vi "main 0.7.vi"() -> ()   [LabVIEW 2012]
uses:
  coherent/CH_LM/CH_LM Communication Mode.ctl
  ISEGNHQxxu/iseg NHQ VISA Control.ctl
  <vilib>/Utility/file.llb/Read From Spreadsheet File (DBL).vi
  <vilib>/Analysis/1siggen.llb/Ramp Pattern by Samples.vi
  <vilib>/Utility/file.llb/Write To Spreadsheet File (DBL).vi
  <vilib>/Utility/file.llb/Write To Spreadsheet File (string).vi
  <vilib>/Platform/browser.llb/Open URL in Default Browser (path).vi
  <vilib>/Analysis/NI_AALBase.lvlib
  coherent/CH_LM.lvlib
panel:
  in  "array size":i32
  out "power noise-o-meter":dbl format="%.1g"
  out "power history":dbl(graph)
  out "signal noise-o-meter":dbl format="%.1g"
  in  "Nominal Voltage":sgl=50.0 max=4000 format="%.2f"
  in  "volt_set":bool
  in  "open base path":bool
  out "laser power":sgl=6.5658234e-09 format="%^#_3e"
  out "Actual Voltage":dbl=-50.050000000000004 format="%.2f"
  out "Waveform Chart":dbl(graph)
  in  "Path":path=path "Y:/Ediff/data/2016/10/161018"
  in  "stop":bool
  out "Slide":dbl(slide)=0.999 scale=0.0..1.0
  in  "Tab Control":T1(tab)
  in  "savepng":bool
  in  "savebin":bool
  in  "dark_load":bool
  in  "binning":dbl=4.0
  in  "exp time [s]":dbl=0.01
  in  "frames":i32=1000
  in  "avg[t] acc[f]":bool=TRUE
  in  "threshold":i32=110
  in  "dark?":bool=TRUE
  in  "dark":bool
  in  "snap":bool
  in  "count?":bool
  in  "move2com":bool
  in  "window2":dbl=10000.0 caption="+/- window" format="%#_6e"
  in  "steps2":u32=21 caption="steps"
  out "XY":dbl[][](graph)
  in  "meas_start_XY":bool
  in  "Axis2":string(combo)="4D Z"
  in  "Axis1":string(combo)="4D Z"
  in  "window1":dbl=10000.0 caption="+/- window" format="%#_6e"
  in  "steps1":u32=21 caption="steps"
  in  "meas_stop_XY":bool
  in  "showcom":bool
  out "Slide 2":dbl(slide)=0.999 scale=0.0..1.0
  in  "meas_stop_volt":bool
  in  "meas_start_volt":bool
  in  "head":string="PowerVoltScan1"
  in  "volt_start":dbl format="%0.2f"
  in  "volt_end":dbl=1.0 format="%0.2f"
  in  "volt_samples":i32=128
  out "Boolean":bool
  out "XY Graph":cluster{sgl[], dbl[]}(graph)
  in  "x .or. y?":bool
  in  "head 2":string="PowerVoltScan1"
  in  "meas_start_power":bool
  in  "VISA ISEG":refnum<visa-resource-name>="COM6"
  in  "Channel (A)":enum16{"A", "B"}(ring)=enum."B"
  in  "IP address":string="172.24.192.135"
  out "error out":errorcluster
  out "coherent":errorcluster
  in  "volt_timeout":u32=6000
  in  "volt_threshold":sgl=2.0 max=4000 format="%.2f"
  out "captured":dbl[][](graph)
  out "live":dbl[][](graph)
  in  "close":bool
  # "%"
  # "%"
  # "V"
  # "W"
  # "Axis2"
  # "Axis1"
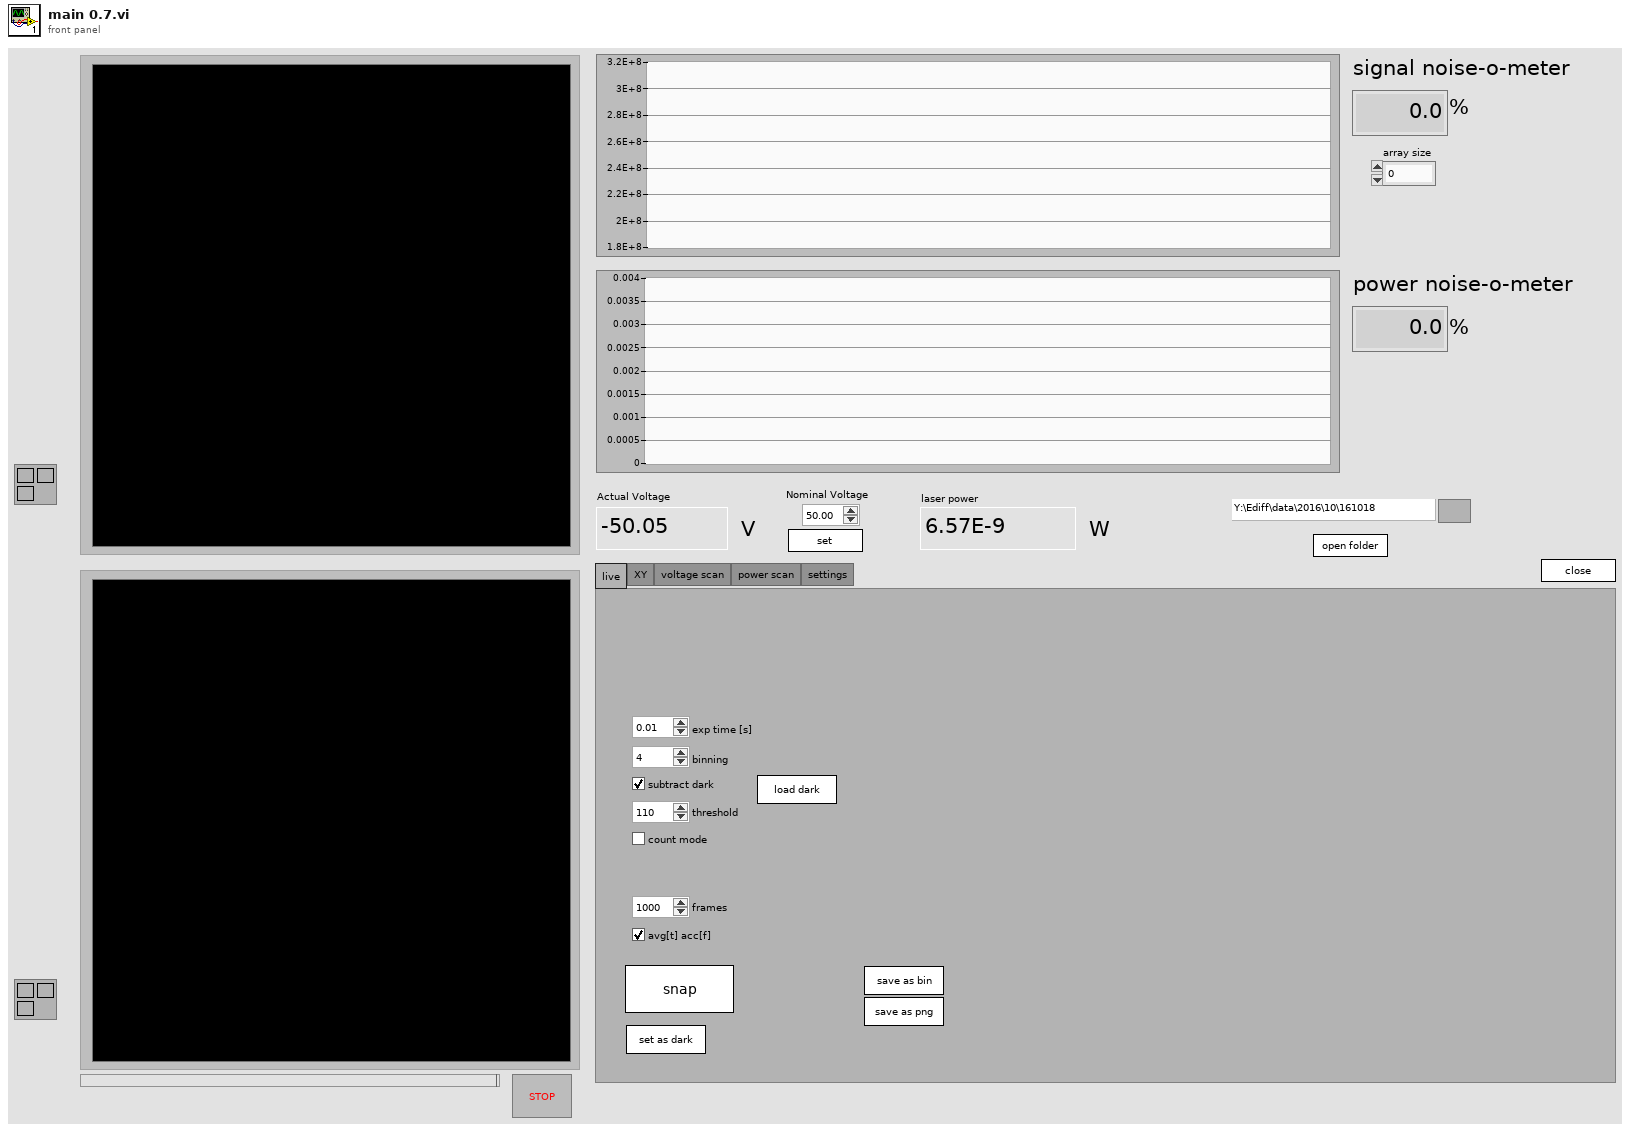
[diagram p1: front panel]
types:
  T1 = enum32{"live", "XY", "voltage scan", "power scan", "settings"}
  T2 = typedef "CH_LM.lvlib/CH_LM Communication Mode.ctl" = enum16{"None", "USB", "GPIB", "RS232"}
  T3 = typedef "Image Type" = u32
  T4 = typedef "IMAQ Image.ctl" = refnum<image>
  T5 = cluster{"height":u32, "width":u32, "datatype":u32}
  T6 = typedef "iseg NHQ VISA Control.ctl" = cluster{"VISA Resource Name":refnum<visa-resource-name>, "FP Notation":bool, "Maximum Voltage":u32, "Maximum Current":u32}
  T7 = typedef "CH_LM.lvlib/CH_LM Streaming Data.ctl" = cluster{"Value":sgl, "Quad Distance":cluster{"X":sgl, "Y":sgl}, "Display Data":cluster{"Format ID":u8, "Scale ID":u8}, "Unit ID":u8, "Flags":u32, "Pulse Period":u32, "Sequence ID":u32, "Unit String":string}
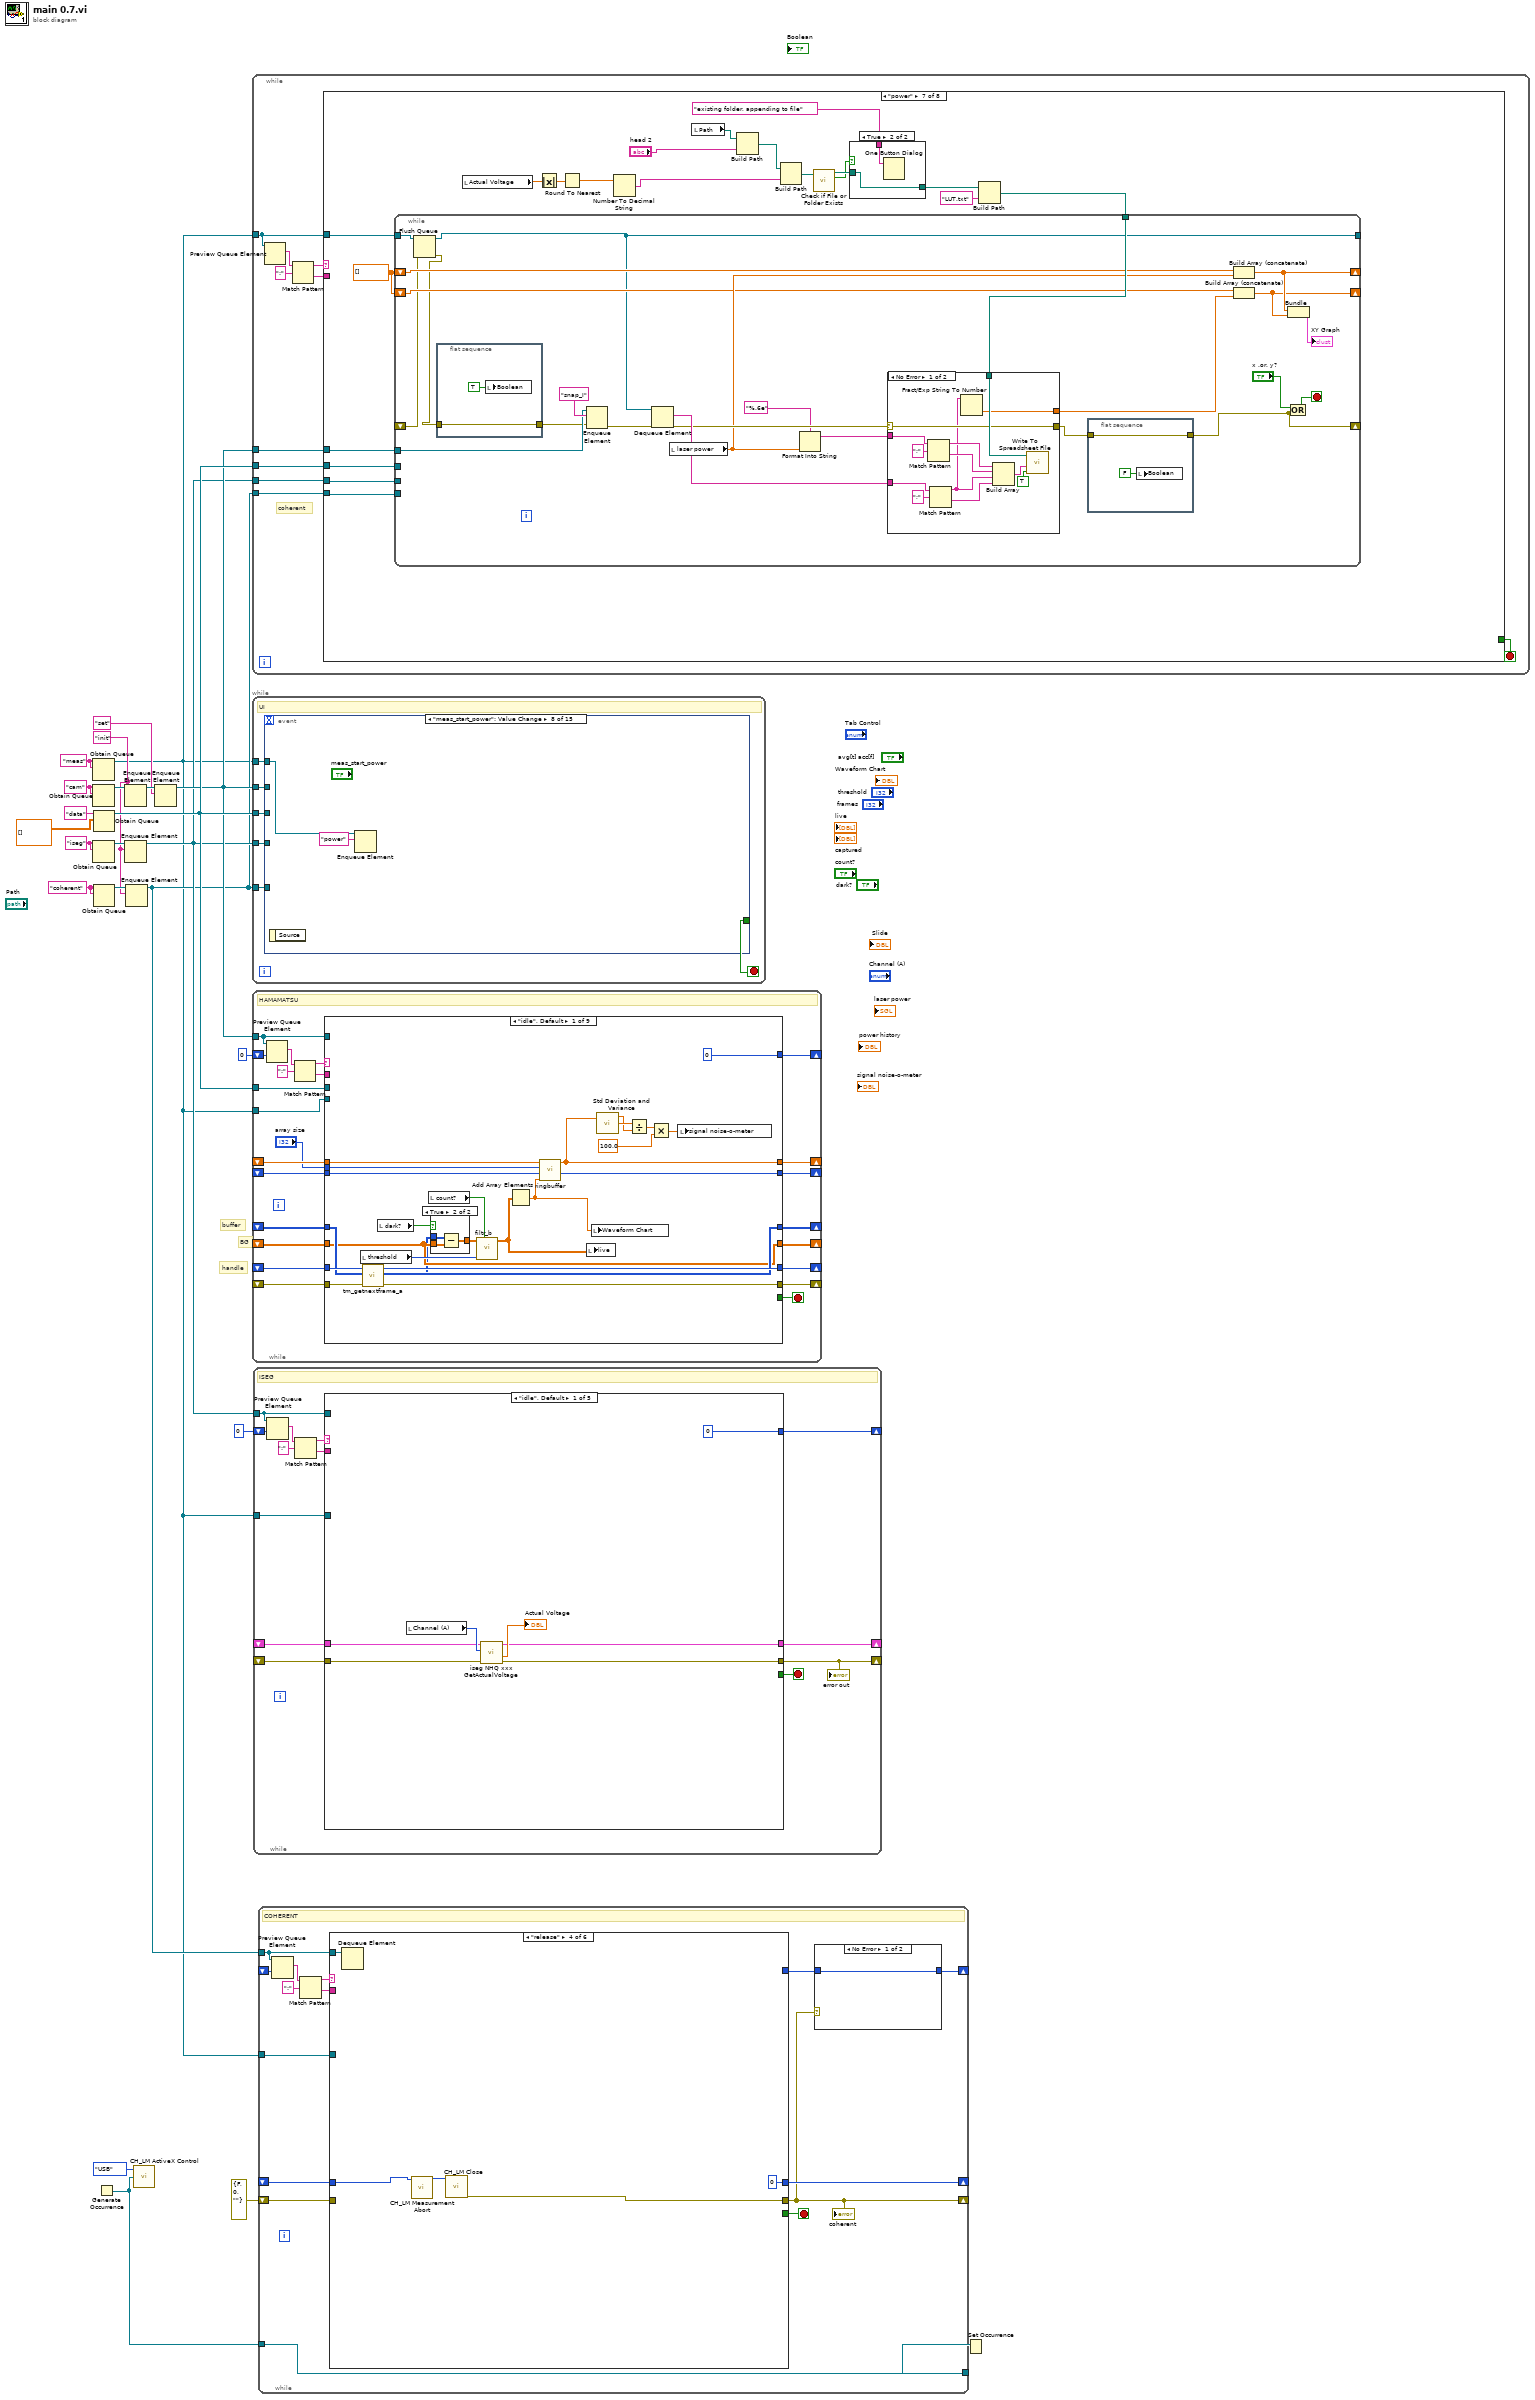
[diagram p0: block diagram]
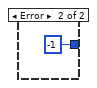
[diagram p2: hidden frame]
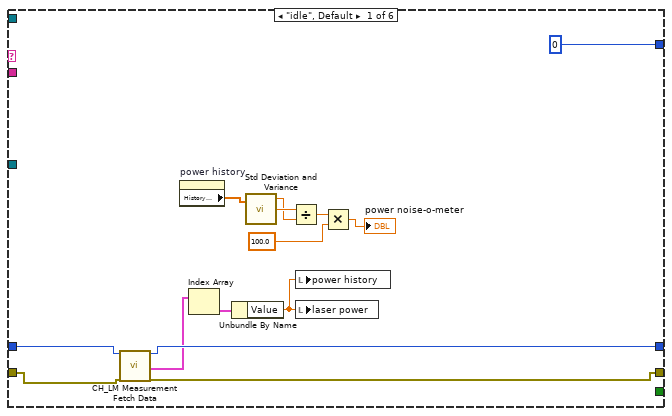
[diagram p3: hidden frame]
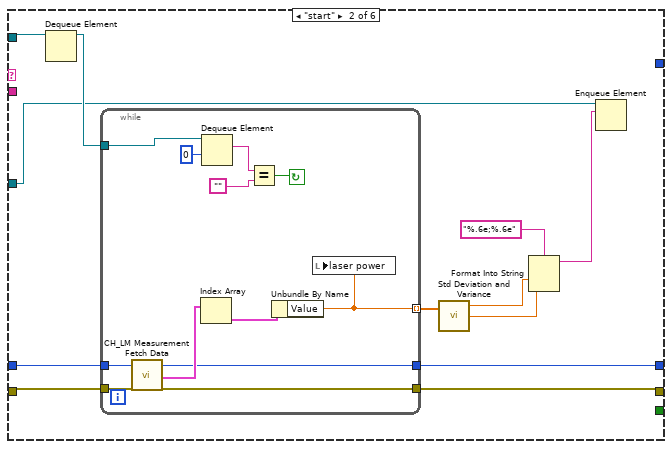
[diagram p4: hidden frame]
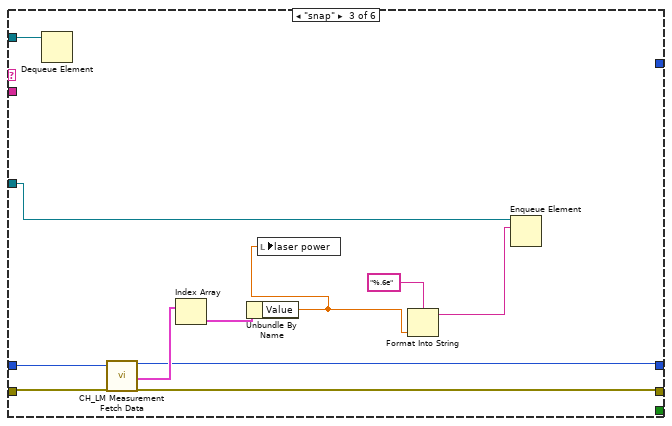
[diagram p5: hidden frame]
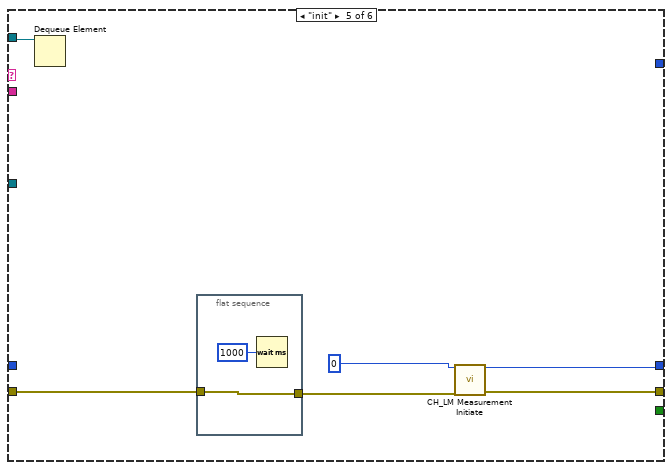
[diagram p6: hidden frame]
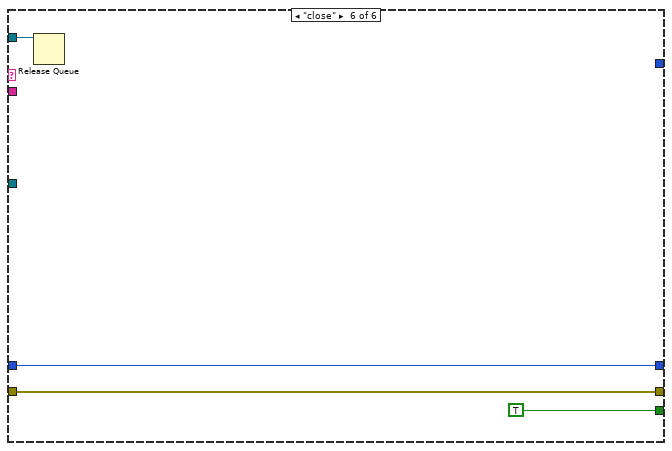
[diagram p7: hidden frame]
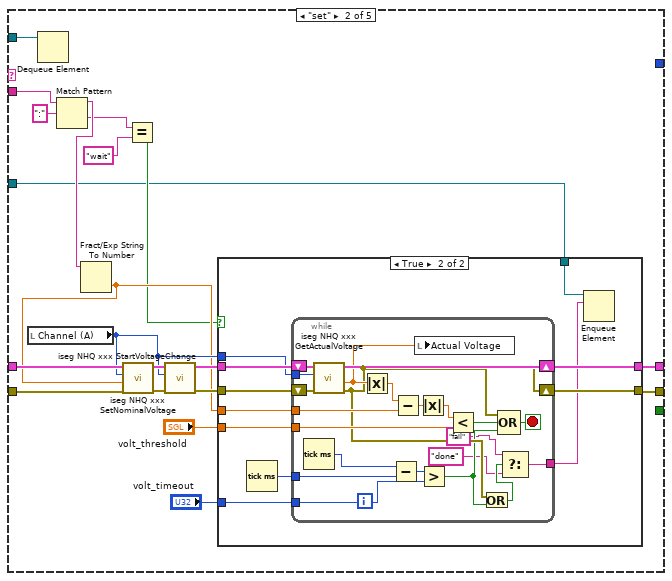
[diagram p8: hidden frame]
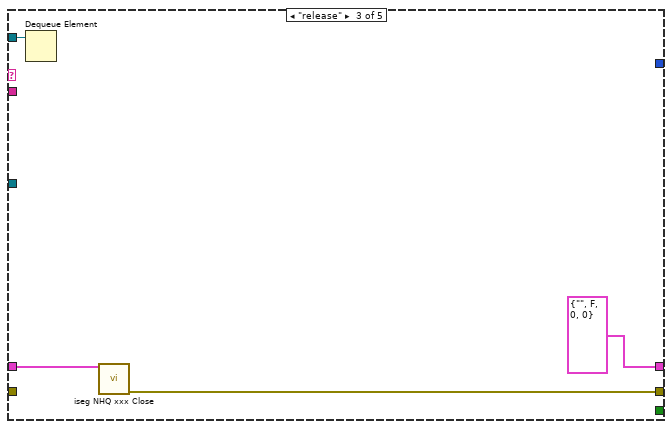
[diagram p10: hidden frame]
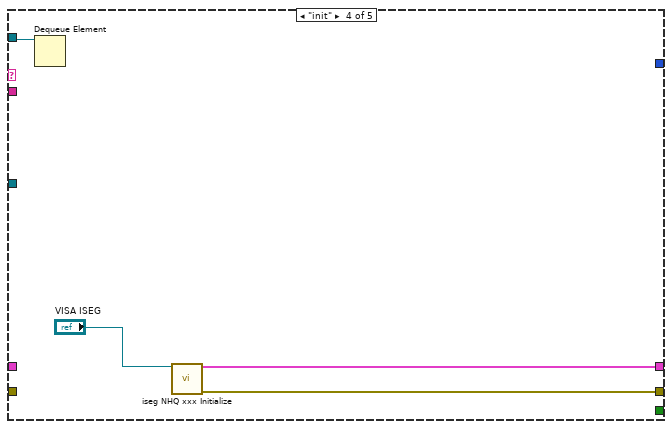
[diagram p11: hidden frame]
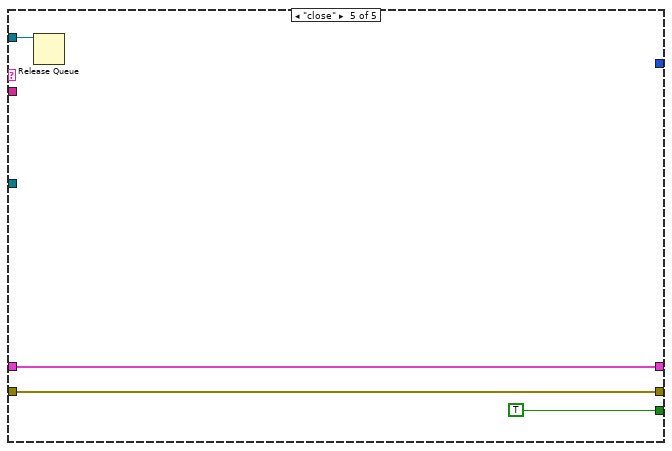
[diagram p12: hidden frame]
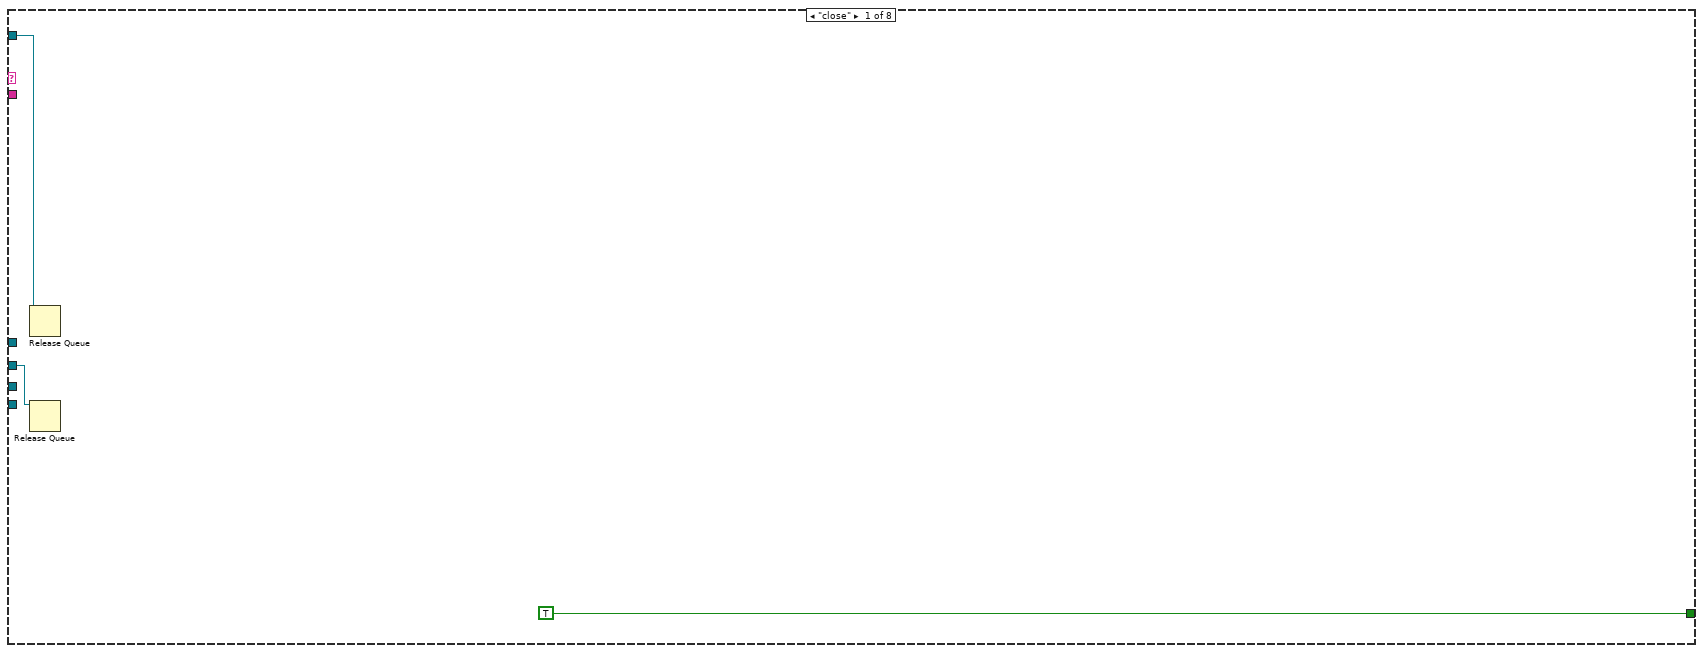
[diagram p13: hidden frame]
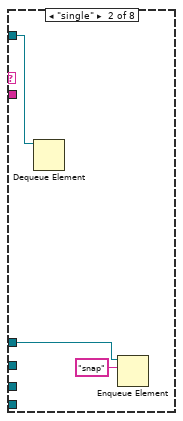
[diagram p14: hidden frame]
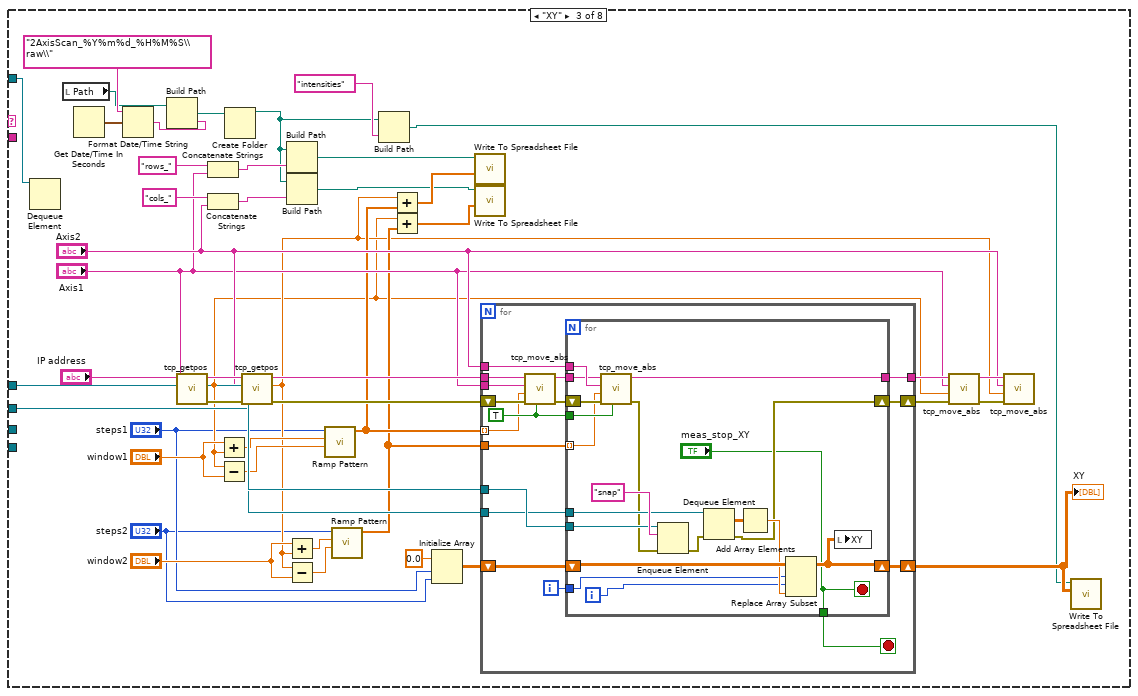
[diagram p15: hidden frame]
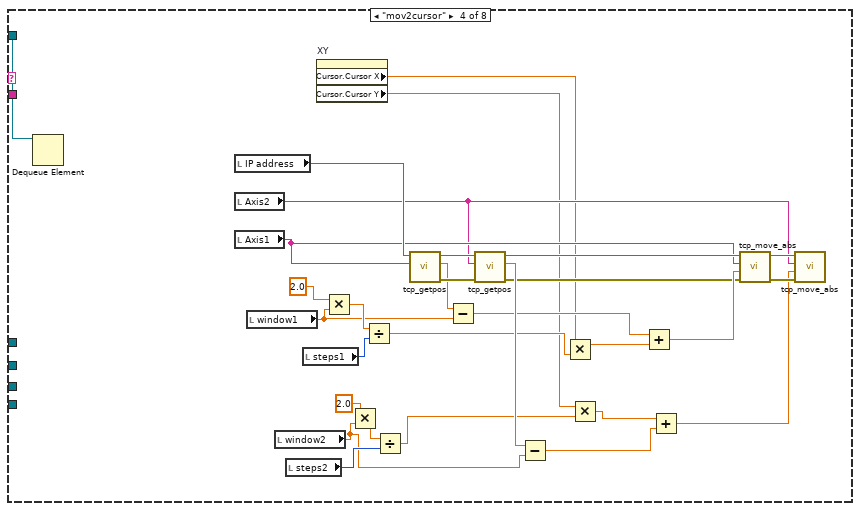
[diagram p16: hidden frame]
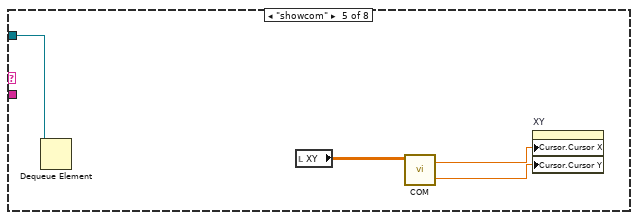
[diagram p17: hidden frame]
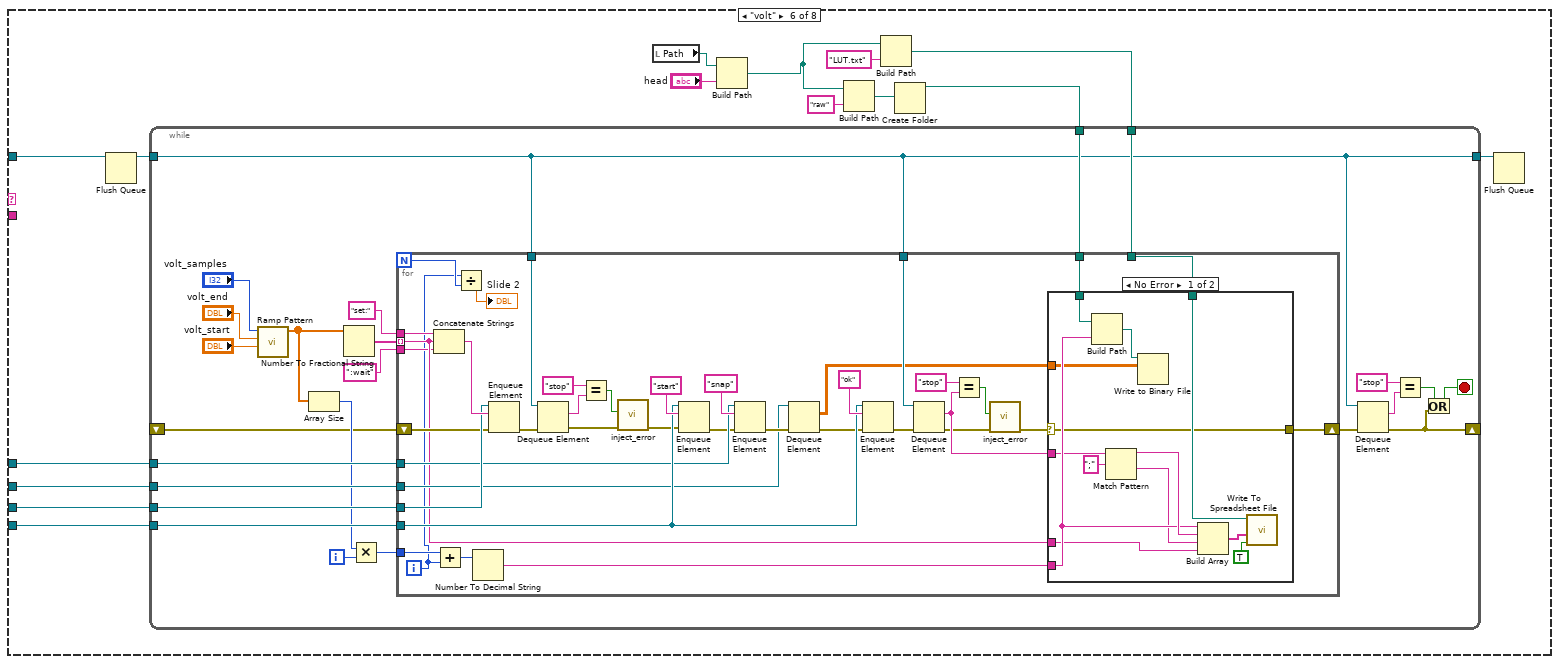
[diagram p18: hidden frame]
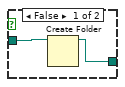
[diagram p20: hidden frame]
diagram:
  w8 = "coherent" ("name (unnamed)")
  w13 = "iseg" ("name (unnamed)")
  w7 = "init" ("element")
  w20 = "meas" ("name (unnamed)")
  w21 = "cam" ("name (unnamed)")
  # "BG"
  # "handle"
  # "buffer"
  n1 = Obtain Queue(name (unnamed)=w20, element data type=w20) -> (queue out=w1:refnum<queue>)  [unwired: 3 in, 2 out]
  n2 = Obtain Queue(name (unnamed)=w21, element data type=w21) -> (queue out=w23:refnum<queue>)  [unwired: 3 in, 2 out]
  n3 = Obtain Queue(name (unnamed)=w13, element data type=w13) -> (queue out=w12:refnum<queue>)  [unwired: 3 in, 2 out]
  n4 = Obtain Queue(name (unnamed)="data", element data type=dbl[][] []) -> (queue out=w16:refnum<queue>)  [unwired: 3 in, 2 out]
  n5 = Obtain Queue(name (unnamed)=w8, element data type=w8) -> (queue out=w9:refnum<queue>)  [unwired: 3 in, 2 out]
  n6 = Generate Occurrence() -> (w5:refnum<k4>)
  n7 = Enqueue Element(queue=w23, element=w7) -> (queue out=w19:refnum<queue>)  [unwired: 2 in, 2 out]
  n8 = Enqueue Element(queue=w12, element=w7) -> (queue out=w10:refnum<queue>)  [unwired: 2 in, 2 out]
  n9 = Enqueue Element(queue=w9, element=w7) -> (queue out=w3:refnum<queue>)  [unwired: 2 in, 2 out]
  n10 = call "CH_LM ActiveX Control.vi"("Communication Mode"=CH_LM_Communication_Mode."USB", "MonitorStop Occurrence"=w5) -> ()  [unwired: 3 in, 1 out]
  n11 = Enqueue Element(queue=w19, element="set") -> (queue out=w15:refnum<queue>)  [unwired: 2 in, 2 out]
  n12 = while {
    tunnel: w1 -> [w29]
    tunnel: w16 -> [w28]
    tunnel: w15 -> [w26]
    tunnel: w10 -> [w25]
    tunnel: w3 -> [w24]
    stop <- w27 stop-if-true
    # "coherent"
    n13 = Preview Queue Element(queue=w29) -> (element=w33:string)  [unwired: 2 in, 3 out]
    n14 = Match Pattern(string=w33, regular expression=":") -> (before substring=w31:string, after substring=w30:string)  [unwired: 1 in, 2 out]
    n15 = case shown="\"power\"" w31 {
      tunnel: w30 -> [_ _ _ _ _ _ _ _]
      tunnel: w29 -> [w35 w39 w84 w150 w151 w169 w257 _]
      tunnel: w28 -> [w36 _ w80 _ _ w161 w264 _]
      tunnel: [TRUE _ _ _ _ _ _ _] -> w27
      tunnel: w26 -> [_ w38 w81 _ _ w162 w265 _]
      tunnel: w25 -> [_ _ _ _ _ w163 w263 _]
      tunnel: w24 -> [_ _ _ _ _ w164 w262 _]
      frame "close" {
        n16 = Release Queue(queue=w35) -> ()  [unwired: 2 in, 3 out]
        n17 = Release Queue(queue=w36) -> ()  [unwired: 2 in, 3 out]
      }
      frame "single" {
        n18 = Dequeue Element(queue=w39) -> ()  [unwired: 2 in, 4 out]
        n19 = Enqueue Element(queue=w38, element="snap") -> ()  [unwired: 2 in, 3 out]
      }
      frame "XY" {
        n20 = Dequeue Element(queue=w84) -> ()  [unwired: 2 in, 4 out]
        n21 = local read "Path"() -> (w75:path)
        n22 = Get Date/Time In Seconds() -> (seconds since 1Jan1904=w79:timestamp)
        n23 = Format Date/Time String(time format string (%c)="2AxisScan_%Y%m%d_%H%M%S\\raw\\", seconds (now)=w79) -> (date/time string=w43:string)  [unwired: 1 in]
        n24 = Build Path(base path=w75, name or relative path=w43) -> (appended path=w47:path)
        n25 = call "tcp_getpos.vi"("Axis"="Axis1", "IP address"="IP address") -> ("error out"=w76:errorcluster, "position"=w52:dbl, "IP address out"=w77:string)  [unwired: 7 in]
        n26 = Concatenate Strings("rows_" ("string"), "Axis1") -> (w44:string)
        n27 = Concatenate Strings("cols_" ("string"), "Axis2") -> (w74:string)
        n28 = Add(x="window1", y=w52) -> (x+y=w59:dbl)
        n29 = Subtract(x=w52, y="window1") -> (x-y=w58:dbl)
        n30 = Create Folder(path (use dialog)=w47) -> (created path=w42:path)  [unwired: 2 in, 2 out]
        n31 = call "tcp_getpos.vi"("error in (no error)"=w76, "Axis"="Axis2", "IP address"=w77) -> ("error out"=w69:errorcluster, "position"=w53:dbl, "IP address out"=w64:string)  [unwired: 6 in]
        n32 = Build Path(base path=w42, name or relative path=w44) -> (appended path=w41:path)
        n33 = Build Path(base path=w42, name or relative path=w74) -> (appended path=w40:path)
        n34 = Add(x="window2", y=w53) -> (x+y=w56:dbl)
        n35 = Subtract(x=w53, y="window2") -> (x-y=w57:dbl)
        n36 = call-poly <vilib>:"Ramp Pattern.vi"("start"=w58, "end"=w59, "samples"="steps1") -> ("Ramp Pattern"=w55:dbl[])  [unwired: 7 in, 1 out]
        n37 = call-poly <vilib>:"Ramp Pattern.vi"("start"=w57, "end"=w56, "samples"="steps2") -> ("Ramp Pattern"=w54:dbl[])  [unwired: 7 in, 1 out]
        n38 = Build Path(base path=w42, name or relative path="intensities") -> (appended path=w45:path)
        n39 = Add(x=w53, y=w55) -> (x+y=w51:dbl[])
        n40 = Add(x=w52, y=w54) -> (x+y=w50:dbl[])
        n41 = Initialize Array(0.0 ("element"), "steps1", "steps2") -> (w82:dbl[][])
        n42 = call-poly <vilib>:"Write To Spreadsheet File.vi"("1D data"=w51, "file path (dialog if empty)"=w41) -> ()  [unwired: 6 in, 1 out]
        n43 = call-poly <vilib>:"Write To Spreadsheet File.vi"("1D data"=w50, "file path (dialog if empty)"=w40) -> ()  [unwired: 6 in, 1 out]
        n44 = for {
          tunnel: "Axis1" -> [w101]
          tunnel: w81 -> [w100]
          tunnel: w80 -> [w99]
          tunnel: "Axis2" -> [w95]
          shift-right: [w94] -> w73
          shift-left: w82 -> [w98]
          shift-right: [w91] -> w70
          shift-left: w69 -> [w90]
          tunnel: [w88] -> w65
          tunnel: w64 -> [w87]
          tunnel: w55 -> [w85] mode=indexing
          tunnel: w54 -> [w86]
          i -> [w97]
          stop <- w89 stop-if-true
          w96 = TRUE ("wait4motiondone")
          n45 = call "tcp_move_abs.vi"("wait4motiondone"=w96, "error in (no error)"=w90, "destination nm/u°"=w85, "Axis"=w101, "IP address"=w87) -> ("error out"=w93:errorcluster, "IP address out"=w92:string)  [unwired: 4 in, 1 out]
          n46 = for {
            tunnel: w100 -> [w118]
            tunnel: w99 -> [w117]
            tunnel: w97 -> [w103]
            shift-right: [w108] -> w94
            shift-left: w98 -> [w116]
            tunnel: w96 -> [w112]
            tunnel: w95 -> [w111]
            tunnel: w92 -> [w109]
            shift-right: [w107] -> w91
            shift-left: w93 -> [w110]
            tunnel: ["meas_stop_XY"] -> w89
            tunnel: [w105] -> w88
            tunnel: w86 -> [w104] mode=indexing
            i -> [w102]
            stop <- "meas_stop_XY" stop-if-true
            n47 = call "tcp_move_abs.vi"("wait4motiondone"=w112, "error in (no error)"=w110, "destination nm/u°"=w104, "Axis"=w111, "IP address"=w109) -> ("error out"=w113:errorcluster, "IP address out"=w105:string)  [unwired: 4 in, 1 out]
            n48 = Enqueue Element(queue=w118, element="snap", error in (no error)=w113) -> (error out=w119:errorcluster)  [unwired: 1 in, 2 out]
            n49 = Dequeue Element(queue=w117, error in (no error)=w119) -> (element=w115:dbl[][], error out=w107:errorcluster)  [unwired: 1 in, 2 out]
            n50 = Add Array Elements(numeric array=w115) -> (sum=w114:dbl)
            n51 = Replace Array Subset(array=w116, new element=w114, index (row)=w103, index (col)=w102) -> (w108:dbl[][])
            n52 = local write "XY"(w108) -> ()
          }
        }
        "XY" <- w73
        n53 = call "tcp_move_abs.vi"("error in (no error)"=w70, "destination nm/u°"=w52, "Axis"="Axis1", "IP address"=w65) -> ("error out"=w72:errorcluster, "IP address out"=w71:string)  [unwired: 5 in, 1 out]
        n54 = call "tcp_move_abs.vi"("error in (no error)"=w72, "destination nm/u°"=w53, "Axis"="Axis2", "IP address"=w71) -> ()  [unwired: 5 in, 3 out]
        n55 = call-poly <vilib>:"Write To Spreadsheet File.vi"("2D data"=w73, "file path (dialog if empty)"=w45) -> ()  [unwired: 6 in, 1 out]
      }
      frame "mov2cursor" {
        n56 = Dequeue Element(queue=w150) -> ()  [unwired: 2 in, 4 out]
        n57 = local read "IP address"() -> (w145:string)
        n58 = local read "Axis2"() -> (w123:string)
        n59 = local read "Axis1"() -> (w124:string)
        n60 = local read "window1"() -> (w138:dbl)
        n61 = local read "window2"() -> (w137:dbl)
        n62 = local read "steps2"() -> (w143:u32)
        n63 = local read "steps1"() -> (w144:u32)
        n64 = property on="XY" class="IntGraph (strict)"() -> ("Cursor.Cursor X"=w122:dbl, "Cursor.Cursor Y"=w121:dbl)  [unwired: 2 in, 2 out]
        n65 = Multiply(x=2.0, y=w138) -> (x*y=w142:dbl)
        n66 = Multiply(x=2.0, y=w137) -> (x*y=w139:dbl)
        n67 = Divide(x=w142, y=w144) -> (x/y=w136:dbl)
        n68 = Divide(x=w139, y=w143) -> (x/y=w133:dbl)
        n69 = call "tcp_getpos.vi"("Axis"=w124, "IP address"=w145) -> ("error out"=w148:errorcluster, "position"=w146:dbl, "IP address out"=w149:string)  [unwired: 7 in]
        n70 = Subtract(x=w146, y=w138) -> (x-y=w134:dbl)
        n71 = call "tcp_getpos.vi"("error in (no error)"=w148, "Axis"=w123, "IP address"=w149) -> ("error out"=w126:errorcluster, "position"=w147:dbl, "IP address out"=w125:string)  [unwired: 6 in]
        n72 = Subtract(x=w147, y=w137) -> (x-y=w131:dbl)
        n73 = Multiply(x=w122, y=w136) -> (x*y=w135:dbl)
        n74 = Multiply(x=w121, y=w133) -> (x*y=w132:dbl)
        n75 = Add(x=w134, y=w135) -> (x+y=w128:dbl)
        n76 = Add(x=w132, y=w131) -> (x+y=w127:dbl)
        n77 = call "tcp_move_abs.vi"("error in (no error)"=w126, "destination nm/u°"=w128, "Axis"=w124, "IP address"=w125) -> ("error out"=w130:errorcluster, "IP address out"=w129:string)  [unwired: 5 in, 1 out]
        n78 = call "tcp_move_abs.vi"("error in (no error)"=w130, "destination nm/u°"=w127, "Axis"=w123, "IP address"=w129) -> ()  [unwired: 5 in, 3 out]
      }
      frame "showcom" {
        n79 = Dequeue Element(queue=w151) -> ()  [unwired: 2 in, 4 out]
        n80 = local read "XY"() -> (w154:dbl[][])
        n81 = call "COM.vi"("Array"=w154) -> ("Y out"=w152:dbl, "X out"=w153:dbl)  [unwired: 3 in]
        n82 = property on="XY" class="IntGraph (strict)"("Cursor.Cursor X"=w153, "Cursor.Cursor Y"=w152) -> ()  [unwired: 2 in, 2 out]
      }
      frame "volt" {
        n83 = Flush Queue(queue=w169) -> (queue out=w165:refnum<queue>)  [unwired: 1 in, 2 out]
        n84 = local read "Path"() -> (w168:path)
        n85 = Build Path(base path=w168, name or relative path="head") -> (appended path=w156:path)
        n86 = Build Path(base path=w156, name or relative path="raw") -> (appended path=w158:path)
        n87 = Build Path(base path=w156, name or relative path="LUT.txt") -> (appended path=w159:path)
        n88 = Create Folder(path (use dialog)=w158) -> (created path=w157:path)  [unwired: 2 in, 2 out]
        n89 = while {
          tunnel: w165 -> [w170]
          tunnel: w164 -> [w193]
          tunnel: w163 -> [w187]
          tunnel: w162 -> [w186]
          tunnel: w161 -> [w185]
          tunnel: w159 -> [w180]
          tunnel: w157 -> [w179]
          shift-right: [w172] -> _
          shift-left: _ -> [w177]
          tunnel: [w170] -> w155
          i -> [w184]
          stop <- w171 stop-if-true
          n90 = call-poly <vilib>:"Ramp Pattern.vi"("start"="volt_start", "end"="volt_end", "samples"="volt_samples") -> ("Ramp Pattern"=w183:dbl[])  [unwired: 7 in, 1 out]
          n91 = Array Size(array=w183) -> (size(s)=w182:i32)
          n92 = Number To Fractional String(number=w183) -> (F-format string=w189:string[])  [unwired: 3 in]
          n93 = Multiply(x=w182, y=w184) -> (x*y=w181:i32)
          n94 = for {
            N -> [w196]
            tunnel: w193 -> [w223]
            tunnel: w170 -> [w230]
            tunnel: w189 -> [w213] mode=indexing
            tunnel: "set:" ("element") -> [w227]
            tunnel: w187 -> [w226]
            tunnel: w170 -> [w224]
            tunnel: w186 -> [w221]
            tunnel: w185 -> [w218]
            shift-right: [w198] -> w178
            shift-left: w177 -> [w216]
            tunnel: w181 -> [w215]
            tunnel: w180 -> [w212]
            tunnel: w179 -> [w211]
            tunnel: ":wait" ("element") -> [w197]
            i -> [w195]
            n95 = Concatenate Strings(w227, w213, w197) -> (w228:string)
            n96 = Add(x=w215, y=w195) -> (x+y=w214:i32)
            n97 = Divide(x=w195, y=w196) -> (x/y=→"Slide 2":dbl)
            n98 = Number To Decimal String(number=w214) -> (decimal integer string=w210:string)  [unwired: 1 in]
            n99 = Enqueue Element(queue=w226, element=w228, error in (no error)=w216) -> (error out=w225:errorcluster)  [unwired: 1 in, 2 out]
            n100 = Dequeue Element(queue=w224, error in (no error)=w225) -> (element=w207:string, error out=w205:errorcluster)  [unwired: 1 in, 2 out]
            n101 = Equal?(x="stop" ("y"), y=w207) -> (x = y?=w204:bool)
            n102 = call "inject_error.vi"("error in"=w205, "s"=w204) -> ("error out"=w206:errorcluster)  [unwired: 9 in]
            n103 = Enqueue Element(queue=w223, element="start", error in (no error)=w206) -> (error out=w220:errorcluster)  [unwired: 1 in, 2 out]
            n104 = Enqueue Element(queue=w221, element="snap", error in (no error)=w220) -> (error out=w219:errorcluster)  [unwired: 1 in, 2 out]
            n105 = Dequeue Element(queue=w218, error in (no error)=w219) -> (element=w209:dbl[][], error out=w217:errorcluster)  [unwired: 1 in, 2 out]
            n106 = Enqueue Element(queue=w223, element="ok", error in (no error)=w217) -> (error out=w229:errorcluster)  [unwired: 1 in, 2 out]
            n107 = Dequeue Element(queue=w230, error in (no error)=w229) -> (element=w201:string, error out=w200:errorcluster)  [unwired: 1 in, 2 out]
            n108 = Equal?(x="stop" ("y"), y=w201) -> (x = y?=w203:bool)
            n109 = call "inject_error.vi"("error in"=w200, "s"=w203) -> ("error out"=w199:errorcluster)  [unwired: 9 in]
            n110 = case shown="No Error" w199 {
              selector: w199 -> [w235 w246]
              tunnel: w213 -> [w234 _]
              tunnel: w212 -> [w241 _]
              tunnel: w211 -> [w240 _]
              tunnel: w210 -> [w239 _]
              tunnel: w209 -> [w237 _]
              tunnel: w201 -> [w236 _]
              tunnel: [w235 w246] -> w198
              frame No Error {
                n111 = Build Path(base path=w240, name or relative path=w239) -> (appended path=w238:path)
                n112 = Match Pattern(string=w236, regular expression=";") -> (before substring=w243:string, after substring=w233:string)  [unwired: 1 in, 2 out]
                n113 = Write to Binary File(file (use dialog)=w238, data=w237) -> ()  [unwired: 4 in, 3 out]
                n114 = Build Array(w239, w243, w233, w234) -> (w242:string[])
                n115 = call-poly <vilib>:"Write To Spreadsheet File.vi"("append to file? (new file:F)"=TRUE, "1D data"=w242, "file path (dialog if empty)"=w241) -> ()  [unwired: 5 in, 1 out]
              }
              frame Error {
              }
            }
          }
          n116 = Dequeue Element(queue=w170, error in (no error)=w178) -> (element=w175:string, error out=w172:errorcluster)  [unwired: 1 in, 2 out]
          n117 = Equal?(x="stop" ("y"), y=w175) -> (x = y?=w173:bool)
          n118 = Or(x=w173, y=w172) -> (x .or. y?=w171:bool)
        }
        n119 = Flush Queue(queue=w155) -> ()  [unwired: 1 in, 3 out]
      }
      frame "power" {
        w258 = sgl[] []
        n120 = local read "Actual Voltage"() -> (w256:dbl)
        n121 = Absolute Value(x=w256) -> (abs(x)=w255:dbl)
        n122 = Round To Nearest(number=w255) -> (nearest integer value=w254:dbl)
        n123 = Number To Decimal String(number=w254) -> (decimal integer string=w253:string)  [unwired: 1 in]
        n124 = local read "Path"() -> (w266:path)
        n125 = Build Path(base path=w266, name or relative path="head 2") -> (appended path=w252:path)
        n126 = Build Path(base path=w252, name or relative path=w253) -> (appended path=w251:path)
        n127 = call <vilib>:"Check if File or Folder Exists.vi"("path"=w251) -> ("file or folder exists?"=w247:bool, "dup path"=w250:path)  [unwired: 8 in, 1 out]
        n128 = case shown="True" w247 {
          tunnel: w250 -> [w268 w270]
          tunnel: [w267 w270] -> w249
          tunnel: "existing folder, appending to file" ("message") -> [_ w269]
          frame False {
            n129 = Create Folder(path (use dialog)=w268) -> (created path=w267:path)  [unwired: 2 in, 2 out]
          }
          frame True {
            n130 = One Button Dialog(message=w269) -> ()  [unwired: 1 in, 1 out]
          }
        }
        n131 = Build Path(base path=w249, name or relative path="LUT.txt") -> (appended path=w260:path)
        n132 = while {
          tunnel: w257 -> [w277]
          tunnel: w262 -> [_]
          tunnel: w263 -> [_]
          tunnel: w265 -> [w286]
          tunnel: w264 -> [_]
          tunnel: w260 -> [w291]
          shift-right: [w274] -> _
          shift-left: _ -> [w271]
          tunnel: [w276] -> _
          shift-right: [w280] -> _
          shift-left: w258 -> [w282]
          shift-right: [w279] -> _
          shift-left: w258 -> [w281]
          stop <- w294 stop-if-true
          n133 = Flush Queue(queue=w277, error in (no error)=w271) -> (queue out=w276:refnum<queue>, error out=w272:errorcluster)  [unwired: 1 out]
          n134 = flat-sequence {
            tunnel: w272 -> [w298]
            tunnel: [w298] -> w273
            frame #0 {
              n135 = local write "Boolean"(TRUE ("Boolean")) -> ()
            }
          }
          n136 = Enqueue Element(queue=w286, element="snap_I", error in (no error)=w273) -> (error out=w292:errorcluster)  [unwired: 1 in, 2 out]
          n137 = Dequeue Element(queue=w276, error in (no error)=w292) -> (element=w290:string, error out=w288:errorcluster)  [unwired: 1 in, 2 out]
          n138 = local read "laser power"() -> (w284:sgl)
          n139 = Format Into String(format string="%.6e", w284) -> (resulting string=w287:string)  [unwired: 2 in, 1 out]
          n140 = case shown="No Error" w288 {
            selector: w288 -> [w306 w313]
            tunnel: w291 -> [w307 _]
            tunnel: [w306 w313] -> w275
            tunnel: w290 -> [w302 _]
            tunnel: w287 -> [w301 _]
            tunnel: [w299 0.0] -> w283
            frame No Error {
              n141 = Match Pattern(string=w301, regular expression=";") -> (before substring=w309:string, after substring=w305:string)  [unwired: 1 in, 2 out]
              n142 = Match Pattern(string=w302, regular expression=";") -> (before substring=w300:string, after substring=w303:string)  [unwired: 1 in, 2 out]
              n143 = Fract/Exp String To Number(string=w300) -> (number=w299:dbl)  [unwired: 3 in, 1 out]
              n144 = Build Array(w309, w305, w300, w303) -> (w308:string[])
              n145 = call-poly <vilib>:"Write To Spreadsheet File.vi"("append to file? (new file:F)"=TRUE, "1D data"=w308, "file path (dialog if empty)"=w307) -> ()  [unwired: 5 in, 1 out]
            }
            frame Error {
            }
          }
          n146 = flat-sequence {
            tunnel: w275 -> [w296]
            tunnel: [w296] -> w274
            frame #0 {
              n147 = local write "Boolean"(FALSE ("Boolean")) -> ()
            }
          }
          n148 = Build Array (concatenate)(w282, w284) -> (w280:sgl[])
          n149 = Build Array (concatenate)(w281, w283) -> (w279:dbl[])
          n150 = Or(x="x .or. y?", y=w274) -> (x .or. y?=w294:bool)
          n151 = Bundle(w280, w279) -> (→"XY Graph":cluster{sgl[], dbl[]})  [unwired: 1 in]
        }
      }
      frame "idle", Default {
      }
    }
  }
  n152 = while {
    tunnel: w15 -> [w319]
    tunnel: w1 -> [w318]
    tunnel: w16 -> [w317]
    tunnel: w10 -> [w315]
    tunnel: w3 -> [w314]
    stop <- w316 stop-if-true
    # "UI"
    n153 = event shown="[7] \"meas_start_power\": Value Change" {
      selector: _ -> [_ _ _ _ _ _ _ _ _ _ _ _ _ _ _]
      dyn-events: _ -> [_ _ _ _ _ _ _ _ _ _ _ _ _ _ _]
      timeout: _ -> [_ _ _ _ _ _ _ _ _ _ _ _ _ _ _]
      tunnel: w319 -> [_ w328 w331 w333 _ _ _ _ _ _ _ w384 _ _ _]
      tunnel: w318 -> [_ w329 _ _ w334 w337 w338 w341 _ _ w378 _ w391 w393 _]
      tunnel: w317 -> [_ _ _ _ _ _ _ _ _ _ _ _ _ _ _]
      tunnel: [_ TRUE _ _ _ _ _ _ _ _ _ _ _ _ _] -> w316
      tunnel: w315 -> [_ w325 _ _ _ _ _ _ _ _ _ _ _ _ w398]
      tunnel: w314 -> [_ w322 _ _ _ _ _ _ _ _ _ _ _ _ _]
      event Timeout {
        n154 = event-data() -> ()  [unwired: 1 in, 1 out]
      }
      event "close": Value Change {
        w320 = "close" ("element")
        w321 = "release" ("element")
        n155 = event-data() -> ()  [unwired: 1 in, 1 out]
        n156 = Enqueue Element(queue=w322, element=w321) -> (queue out=w323:refnum<queue>)  [unwired: 2 in, 2 out]
        n157 = Enqueue Element(queue=w325, element=w321) -> (queue out=w324:refnum<queue>)  [unwired: 2 in, 2 out]
        n158 = Enqueue Element(queue=w328, element=w321) -> (queue out=w327:refnum<queue>)  [unwired: 2 in, 2 out]
        n159 = Enqueue Element(queue=w323, element=w320) -> ()  [unwired: 2 in, 3 out]
        n160 = Enqueue Element(queue=w324, element=w320) -> ()  [unwired: 2 in, 3 out]
        n161 = Enqueue Element(queue=w329, element=w320) -> ()  [unwired: 2 in, 3 out]
        n162 = Enqueue Element(queue=w327, element=w320) -> ()  [unwired: 2 in, 3 out]
      }
      event "dark": Value Change {
        n163 = event-data() -> ()  [unwired: 1 in, 1 out]
        n164 = Enqueue Element(queue=w331, element="dark") -> ()  [unwired: 2 in, 3 out]
      }
      event "binning", "exp time [s]": Value Change {
        n165 = event-data() -> ()  [unwired: 1 in, 1 out]
        n166 = Enqueue Element(queue=w333, element="set") -> ()  [unwired: 2 in, 3 out]
      }
      event "snap": Value Change {
        n167 = event-data() -> ()  [unwired: 1 in, 1 out]
        n168 = Enqueue Element(queue=w334, element="single") -> ()  [unwired: 2 in, 3 out]
      }
      event "meas_start_volt": Value Change {
        n169 = event-data() -> ()  [unwired: 1 in, 1 out]
        n170 = Enqueue Element(queue=w337, element="volt") -> ()  [unwired: 2 in, 3 out]
      }
      event "meas_stop_volt": Value Change {
        n171 = event-data() -> ()  [unwired: 1 in, 1 out]
        n172 = Enqueue Element(queue=w338, element="stop") -> ()  [unwired: 2 in, 3 out]
      }
      event "meas_start_power": Value Change {
        n173 = event-data() -> ()  [unwired: 1 in, 1 out]
        n174 = Enqueue Element(queue=w341, element="power") -> ()  [unwired: 2 in, 3 out]
      }
      event "open base path": Value Change {
        n175 = event-data() -> ()  [unwired: 1 in, 1 out]
        n176 = local read "Path"() -> (w342:path)
        n177 = call-poly <vilib>:"Open URL in Default Browser.vi"("path"=w342) -> ()  [unwired: 5 in, 2 out]
      }
      event "savebin", "savepng": Value Change {
        n178 = event-data() -> ()  [unwired: 1 in, 1 out]
        n179 = Get Date/Time In Seconds() -> (seconds since 1Jan1904=w348:timestamp)
        n180 = local read "Path"() -> (w344:path)
        n181 = Format Date/Time String(time format string (%c)="MCPIMG_%Y%m%d_%H%M%S", seconds (now)=w348) -> (date/time string=w343:string)  [unwired: 1 in]
        n182 = local read "captured"() -> (w345:dbl[][])
        n183 = case shown="False" "savebin" {
          tunnel: w345 -> [w361 w377]
          tunnel: w344 -> [w358 w371]
          tunnel: w343 -> [w356 w372]
          frame False {
            w366 = T3 7 items=["Grayscale (U8)", "Grayscale (I16)", "Grayscale (SGL)", "Complex (CSG)", "RGB (U32)", "HSL (U32)", "RGB (U64)", "Grayscale (U16)"] ("Image Type")
            n184 = for {
              tunnel: w361 -> [w369] mode=indexing
              tunnel: [w368] -> w360 mode=indexing
              n185 = Reverse 1D Array(array=w369) -> (reversed array=w368:dbl[])
            }
            n186 = Concatenate Strings(w356, ".png" ("string")) -> (w357:string)
            n187 = Transpose 2D Array(2D array=w360) -> (transposed array=w351:dbl[][])
            n188 = Build Path(base path=w358, name or relative path=w357) -> (appended path=w359:path)
            n189 = call "IMAQ Create"("Image Name"="untitled", "Image Type"=w366) -> ("New Image"=w367:T4)  [unwired: 3 in, 1 out]
            n190 = Array Max & Min(array=w351) -> (max value=w354:dbl)  [unwired: 3 out]
            n191 = Divide(x=w351, y=w354) -> (x/y=w353:dbl[][])
            n192 = Multiply(x=w353, y=255) -> (x*y=w350:dbl[][])
            n193 = To Unsigned Word Integer(number=w350) -> (unsigned 16bit integer=w349:u16[][])
            n194 = call "IMAQ ArrayToImage"("Image Pixels (U16)"=w349, "Image"=w367) -> ("Image Out"=w365:T4)  [unwired: 8 in, 1 out]
            n195 = call-poly "IMAQ Write File 2"("Image Quality"=u32 1000, "File Path"=w359, "Image"=w365) -> ("Image Out (duplicate)"=w363:T4)  [unwired: 7 in, 1 out]
            n196 = call "IMAQ Dispose"("Image"=w363) -> ()  [unwired: 5 in, 1 out]
          }
          frame True {
            n197 = Concatenate Strings(w372, ".bin" ("string")) -> (w374:string)
            n198 = Build Path(base path=w371, name or relative path=w374) -> (appended path=w370:path)
            n199 = Write to Binary File(file (use dialog)=w370, data=w377) -> (refnum out=w376:refnum<file>, error out=w375:errorcluster)  [unwired: 4 in, 1 out]
            n200 = Close File(refnum=w376, error in=w375) -> ()  [unwired: 2 out]
          }
        }
      }
      event "meas_start_XY": Value Change {
        n201 = event-data() -> ()  [unwired: 1 in, 1 out]
        n202 = Enqueue Element(queue=w378, element="XY") -> ()  [unwired: 2 in, 3 out]
      }
      event "dark_load": Value Change {
        n203 = event-data() -> ()  [unwired: 1 in, 1 out]
        n204 = local read "Path"() -> (w383:path)
        n205 = call "File Dialog"("start path"=w383) -> ("selected path"=w381:path, "cancelled"=w380:bool)  [unwired: 11 in, 2 out]
        n206 = case shown="False" w380 {
          tunnel: w384 -> [w389 _]
          tunnel: "dark_load:" ("element") -> [w387 _]
          tunnel: w381 -> [w385 _]
          frame False {
            n207 = Path To String(path=w385) -> (string=w386:string)
            n208 = Concatenate Strings(w387, w386) -> (w388:string)
            n209 = Enqueue Element(queue=w389, element=w388) -> ()  [unwired: 2 in, 3 out]
          }
          frame True {
          }
        }
      }
      event "move2com": Value Change {
        n210 = event-data() -> ()  [unwired: 1 in, 1 out]
        n211 = Enqueue Element(queue=w391, element="mov2cursor") -> ()  [unwired: 2 in, 3 out]
      }
      event "showcom": Value Change {
        n212 = event-data() -> ()  [unwired: 1 in, 1 out]
        n213 = Enqueue Element(queue=w393, element="showcom") -> ()  [unwired: 2 in, 3 out]
      }
      event "volt_set": Value Change {
        n214 = event-data() -> ()  [unwired: 1 in, 1 out]
        n215 = Number To Fractional String(number="Nominal Voltage") -> (F-format string=w394:string)  [unwired: 3 in]
        n216 = Concatenate Strings("set:" ("element"), w394) -> (w397:string)
        n217 = Enqueue Element(queue=w398, element=w397) -> ()  [unwired: 2 in, 3 out]
      }
    }
  }
  n218 = while {
    tunnel: w15 -> [w417]
    shift-right: [w415] -> _
    shift-left: _ -> [w414]
    shift-right: [w413] -> _
    shift-left: _ -> [w412]
    shift-right: [w411] -> _
    shift-left: _ -> [w410]
    shift-right: [w409] -> _
    shift-left: _ -> [w408]
    shift-right: [w406] -> _
    shift-left: 0 -> [w407]
    tunnel: w16 -> [w405]
    tunnel: w1 -> [w404]
    shift-right: [w403] -> _
    shift-left: _ -> [w402]
    shift-right: [w400] -> _
    shift-left: _ -> [w401]
    stop <- w416 stop-if-true
    # "HAMAMATSU"
    n219 = Preview Queue Element(queue=w417, timeout in ms (-1)=w407) -> (element=w421:string)  [unwired: 1 in, 3 out]
    n220 = Match Pattern(string=w421, regular expression=":") -> (before substring=w419:string, after substring=w418:string)  [unwired: 1 in, 2 out]
    n221 = case shown="\"idle\", Default" w419 {
      tunnel: w418 -> [_ _ _ _ w577 _ _ _ _]
      tunnel: w417 -> [_ w460 w522 w571 w581 w593 w596 w610 w641]
      tunnel: [_ _ _ _ _ _ _ _ TRUE] -> w416
      tunnel: [w440 w462 w527 w569 w578 w585 w601 w611 w636] -> w415
      tunnel: w414 -> [w442 w465 w529 w569 w578 w589 _ w633 w636]
      tunnel: [w441 w457 w526 w568 w579 u32 0 ("Handle out") w599 w612 w637] -> w413
      tunnel: w412 -> [w443 w463 w530 w568 w579 w590 _ w631 w637]
      tunnel: [w439 w464 w525 w570 w580 w591 w597 w613 w638] -> w411
      tunnel: w410 -> [w439 w464 w525 w570 w580 w591 w597 _ w638]
      tunnel: [w438 w461 w528 w567 w574 w592 w598 w614 w639] -> w409
      tunnel: w408 -> [w438 w461 w528 _ _ w592 w598 _ w639]
      tunnel: [0 _ _ _ _ _ _ _ _] -> w406
      tunnel: w405 -> [_ w456 _ _ _ _ _ _ _]
      tunnel: w404 -> [_ _ w523 _ _ _ _ _ _]
      tunnel: [w422 w451 w514 w566 w573 w583 w595 w604 w635] -> w403
      tunnel: w402 -> [w432 w454 w517 w566 w573 w583 w595 w604 w635]
      tunnel: w401 -> [w426 w453 w515 w565 w572 w582 w594 w603 w634]
      tunnel: [w425 w450 w513 w565 w572 w582 w594 w603 w634] -> w400
      tunnel: "array size" -> [w424 w452 w516 _ _ _ _ _ _]
      frame "idle", Default {
        n222 = local read "threshold"() -> (w444:i32)
        n223 = call "tm_getnextframe_a.vi"("error in (no error)"=w442, "Buffer"=w439, "Handle in"=w443) -> ("error out"=w440:errorcluster, "Data"=w434:u16[][], "Handle out"=w441:u32)  [unwired: 6 in]
        n224 = local read "dark?"() -> (w445:bool)
        n225 = local read "count?"() -> (w435:bool)
        n226 = case shown="True" w445 {
          tunnel: [w446 w449] -> w436
          tunnel: w434 -> [w446 w448]
          tunnel: w438 -> [_ w447]
          frame False {
          }
          frame True {
            n227 = Subtract(x=w448, y=w447) -> (x-y=w449:dbl[][])
          }
        }
        n228 = call "filtr_b.vi"("count?"=w435, "threshold"=w444, "input array"=w436) -> ("output array"=w433:dbl[][])  [unwired: 8 in]
        n229 = Add Array Elements(numeric array=w433) -> (sum=w431:dbl)
        n230 = call "ringbuffer.vi"("new val"=w431, "index in"=w426, "array size"=w424, "array in"=w432) -> ("index out"=w425:i32, "array out"=w422:dbl[])  [unwired: 6 in]
        n231 = local write "live"(w433) -> ()
        n232 = local write "Waveform Chart"(w431) -> ()
        n233 = call <vilib>:"Std Deviation and Variance.vi"("X"=w422) -> ("mean"=w427:dbl, "standard deviation"=w430:dbl)  [unwired: 1 in, 1 out]
        n234 = Divide(x=w430, y=w427) -> (x/y=w429:dbl)
        n235 = Multiply(x=w429, y=100.0) -> (x*y=w423:dbl)
        n236 = local write "signal noise-o-meter"(w423) -> ()
      }
      frame "snap" {
        n237 = Dequeue Element(queue=w460) -> ()  [unwired: 2 in, 4 out]
        n238 = local read "avg[t] acc[f]"() -> (w459:bool)
        n239 = local read "threshold"() -> (w467:i32)
        n240 = local read "frames"() -> (w466:i32)
        n241 = local read "count?"() -> (w458:bool)
        n242 = local read "dark?"() -> (w468:bool)
        n243 = for {
          N: w466 -> [w484]
          tunnel: w468 -> [w498]
          tunnel: w464 -> [w496]
          tunnel: w463 -> [w497]
          tunnel: w467 -> [w490]
          tunnel: [w494] -> w457
          shift-right: [w493] -> w462
          shift-left: w465 -> [w495]
          tunnel: w461 -> [w489]
          shift-right: [w483] -> w455
          shift-left: w464 -> [w487]
          tunnel: w459 -> [w488]
          tunnel: w458 -> [w486]
          shift-right: [w475] -> w451
          shift-left: w454 -> [w476]
          tunnel: w452 -> [w473]
          shift-right: [w472] -> w450
          shift-left: w453 -> [w474]
          i -> [w485]
          stop <- "stop" stop-if-true
          n244 = call "tm_getnextframe_a.vi"("error in (no error)"=w495, "Buffer"=w496, "Handle in"=w497) -> ("error out"=w493:errorcluster, "Data"=w492:u16[][], "Handle out"=w494:u32)  [unwired: 6 in]
          n245 = Divide(x=w485, y=w484) -> (x/y=w481:dbl)
          n246 = case shown="True" w498 {
            tunnel: [w509 w512] -> w491
            tunnel: w492 -> [w509 w511]
            tunnel: w489 -> [_ w510]
            frame False {
            }
            frame True {
              n247 = Subtract(x=w511, y=w510) -> (x-y=w512:dbl[][])
            }
          }
          n248 = local write "Slide"(w481) -> ()
          n249 = call "filtr_b.vi"("count?"=w486, "threshold"=w490, "input array"=w491) -> ("output array"=w482:dbl[][])  [unwired: 8 in]
          n250 = Add Array Elements(numeric array=w482) -> (sum=w471:dbl)
          n251 = call "ringbuffer.vi"("new val"=w471, "index in"=w474, "array size"=w473, "array in"=w476) -> ("index out"=w472:i32, "array out"=w475:dbl[])  [unwired: 6 in]
          n252 = call <vilib>:"Std Deviation and Variance.vi"("X"=w475) -> ("mean"=w477:dbl, "standard deviation"=w479:dbl)  [unwired: 1 in, 1 out]
          n253 = local write "live"(w482) -> ()
          n254 = local write "Waveform Chart"(w471) -> ()
          n255 = Divide(x=w479, y=w477) -> (x/y=w470:dbl)
          n256 = case shown="True" w488 {
            tunnel: w487 -> [w501 w508]
            tunnel: w482 -> [w500 w506]
            tunnel: [w499 w502] -> w483
            tunnel: w485 -> [_ w503]
            frame False {
              n257 = Add(x=w501, y=w500) -> (x+y=w499:dbl[][])
            }
            frame True {
              n258 = Multiply(x=w508, y=w503) -> (x*y=w507:dbl[][])
              n259 = Increment(x=w503) -> (x+1=w504:i32)
              n260 = Add(x=w507, y=w506) -> (x+y=w505:dbl[][])
              n261 = Divide(x=w505, y=w504) -> (x/y=w502:dbl[][])
            }
          }
          n262 = local write "captured"(w483) -> ()
          n263 = Multiply(x=w470, y=100.0) -> (x*y=w469:dbl)
          n264 = local write "signal noise-o-meter"(w469) -> ()
        }
        n265 = local write "captured"(w455) -> ()
        n266 = Enqueue Element(queue=w456, element=w455) -> ()  [unwired: 2 in, 3 out]
      }
      frame "snap_I" {
        n267 = Dequeue Element(queue=w522) -> ()  [unwired: 2 in, 4 out]
        n268 = local read "threshold"() -> (w533:i32)
        n269 = local read "frames"() -> (w532:i32)
        n270 = local read "count?"() -> (w531:bool)
        n271 = local read "dark?"() -> (w534:bool)
        n272 = for {
          N: w532 -> [w548]
          tunnel: w534 -> [w560]
          tunnel: w525 -> [w558]
          tunnel: w530 -> [w559]
          tunnel: w533 -> [w552]
          tunnel: [w556] -> w526
          shift-right: [w555] -> w527
          shift-left: w529 -> [w557]
          tunnel: w528 -> [w551]
          tunnel: w531 -> [w550]
          tunnel: [w546] -> w524 mode=indexing
          shift-right: [w538] -> w514
          shift-left: w517 -> [w539]
          tunnel: w516 -> [w537]
          shift-right: [w535] -> w513
          shift-left: w515 -> [w536]
          i -> [w549]
          n273 = call "tm_getnextframe_a.vi"("error in (no error)"=w557, "Buffer"=w558, "Handle in"=w559) -> ("error out"=w555:errorcluster, "Data"=w554:u16[][], "Handle out"=w556:u32)  [unwired: 6 in]
          n274 = call "ringbuffer.vi"("index in"=w536, "array size"=w537, "array in"=w539) -> ("index out"=w535:i32, "array out"=w538:dbl[])  [unwired: 7 in]
          n275 = Divide(x=w549, y=w548) -> (x/y=w547:dbl)
          n276 = case shown="True" w560 {
            tunnel: [w561 w564] -> w553
            tunnel: w554 -> [w561 w563]
            tunnel: w551 -> [_ w562]
            frame False {
            }
            frame True {
              n277 = Subtract(x=w563, y=w562) -> (x-y=w564:dbl[][])
            }
          }
          n278 = local write "Slide"(w547) -> ()
          n279 = call <vilib>:"Std Deviation and Variance.vi"("X"=w538) -> ("mean"=w540:dbl, "standard deviation"=w543:dbl)  [unwired: 1 in, 1 out]
          n280 = call "filtr_b.vi"("count?"=w550, "threshold"=w552, "input array"=w553) -> ("output array"=w545:dbl[][])  [unwired: 8 in]
          n281 = Divide(x=w543, y=w540) -> (x/y=w542:dbl)
          n282 = local write "live"(w545) -> ()
          n283 = Multiply(x=w542, y=100.0) -> (x*y=w544:dbl)
          n284 = local write "signal noise-o-meter"(w544) -> ()
          n285 = Add Array Elements(numeric array=w545) -> (sum=w546:dbl)
          n286 = local write "Waveform Chart"(w546) -> ()
        }
        n287 = call <vilib>:"Std Deviation and Variance.vi"("X"=w524) -> ("mean"=w521:dbl, "standard deviation"=w520:dbl)  [unwired: 1 in, 1 out]
        n288 = Format Into String(format string="%.6e;%.6e", w521, w520) -> (resulting string=w519:string)  [unwired: 2 in, 1 out]
        n289 = Enqueue Element(queue=w523, element=w519) -> ()  [unwired: 2 in, 3 out]
      }
      frame "dark" {
        n290 = Dequeue Element(queue=w571) -> ()  [unwired: 2 in, 4 out]
        n291 = local read "captured"() -> (w567:dbl[][])
      }
      frame "dark_load" {
        n292 = Dequeue Element(queue=w581) -> ()  [unwired: 2 in, 4 out]
        n293 = String To Path(string=w577) -> (path=w576:path)
        n294 = Read from Binary File(5:dbl[][] [] ("all rows"), 11:w576) -> (2:w574:dbl[][])  [unwired: 4 in, 3 out]
        n295 = call-poly <vilib>:"Read From Spreadsheet File.vi"("file path (dialog if empty)"=w576) -> ()  [unwired: 6 in, 5 out]
      }
      frame "release" {
        n296 = call "tm_stopcapture.vi"("error in (no error)"=w589, "Handle in"=w590) -> ("error out"=w587:errorcluster, "Handle out"=w588:u32)  [unwired: 8 in]
        n297 = Dequeue Element(queue=w593) -> ()  [unwired: 2 in, 4 out]
        n298 = call "tm_closecamera.vi"("error in (no error)"=w587, "Handle in"=w588) -> ("error out"=w586:errorcluster)  [unwired: 9 in]
        n299 = call "tm_deinitialize.vi"("error in (no error)"=w586) -> ("error out"=w585:errorcluster)  [unwired: 10 in]
      }
      frame "init" {
        n300 = Dequeue Element(queue=w596) -> ()  [unwired: 2 in, 4 out]
        n301 = call "tm_initialize.vi"() -> ("error out"=w602:errorcluster)  [unwired: 8 in, 3 out]
        n302 = call "tm_opencamera.vi"("error in (no error)"=w602, "Camera Index"=u32 0) -> ("error out"=w601:errorcluster, "Handle out"=w599:u32)  [unwired: 7 in, 1 out]
      }
      frame "set" {
        w619 = 1 items=["Snap", "Sequence"] ("Capture mode")
        w623 = u32 4215968 items=["BINNING"=4215968, "BITS PER CHANNEL"=2, "ACTIVE VIEW INDEX"=3, "CCD MODE"=4, "SENSOR MODE"=5, "READOUT MODE"=6, "EXPOSURE TIME"=7, "CONTRAST GAIN"=8, "CONTRAST OFFSET"=9, "LIGHT MODE"=10, "SENSITIVITY"=11, "WHITE BALANCE"=12, "PHOTON IMAGING MODE"=13, "HIGH DYNAMIC RANGE MODE"=14, "TRIGGER SOURCE"=15, "TRIGGER ACTIVE"=16, "TRIGGER MODE"=17, "TRIGGER POLARITY"=18, "TRIGGER GLOBAL EXPOSURE"=19, "FIRST TRIGGER BEHAVIOR"=20, "TRIGGER TIMES"=21, "OUTPUT TRIGGER POLARITY"=22, "OUTPUT TRIGGER DELAY"=23, "OUTPUT TRIGGER PERIOD"=24, "TEMPERATURE"=25, "TEMPERATURE TARGET"=26, "SENSOR COOLER FAN"=27, "MECHANICAL SHUTTER"=28, "BACK FOCUS POSITION"=29, "FRAMEBUNDLE MODE"=30, "FRAMEBUNDLE NUMBER"=31, "LINEBUNDLE HEIGHT"=32, "TRIGGER CONNECTOR"=33, "IMAGE PIXEL TYPE"=34, "OUTPUT TRIGGER KIND"=35, "READOUT DIRECTION"=36, "CHANNEL SYNC"=37] ("Parameter")
        w627 = u32 7 items=["BINNING"=4215968, "BITS PER CHANNEL"=2, "ACTIVE VIEW INDEX"=3, "CCD MODE"=4, "SENSOR MODE"=5, "READOUT MODE"=6, "EXPOSURE TIME"=7, "CONTRAST GAIN"=8, "CONTRAST OFFSET"=9, "LIGHT MODE"=10, "SENSITIVITY"=11, "WHITE BALANCE"=12, "PHOTON IMAGING MODE"=13, "HIGH DYNAMIC RANGE MODE"=14, "TRIGGER SOURCE"=15, "TRIGGER ACTIVE"=16, "TRIGGER MODE"=17, "TRIGGER POLARITY"=18, "TRIGGER GLOBAL EXPOSURE"=19, "FIRST TRIGGER BEHAVIOR"=20, "TRIGGER TIMES"=21, "OUTPUT TRIGGER POLARITY"=22, "OUTPUT TRIGGER DELAY"=23, "OUTPUT TRIGGER PERIOD"=24, "TEMPERATURE"=25, "TEMPERATURE TARGET"=26, "SENSOR COOLER FAN"=27, "MECHANICAL SHUTTER"=28, "BACK FOCUS POSITION"=29, "FRAMEBUNDLE MODE"=30, "FRAMEBUNDLE NUMBER"=31, "LINEBUNDLE HEIGHT"=32, "TRIGGER CONNECTOR"=33, "IMAGE PIXEL TYPE"=34, "OUTPUT TRIGGER KIND"=35, "READOUT DIRECTION"=36, "CHANNEL SYNC"=37] ("Parameter")
        n303 = Dequeue Element(queue=w610) -> ()  [unwired: 2 in, 4 out]
        n304 = call "tm_stopcapture.vi"("error in (no error)"=w633, "Handle in"=w631) -> ("error out"=w632:errorcluster, "Handle out"=w630:u32)  [unwired: 8 in]
        n305 = call "tm_unpreparecapture.vi"("error in (no error)"=w632, "Handle in"=w630) -> ("error out"=w629:errorcluster, "Handle out"=w628:u32)  [unwired: 8 in]
        n306 = call "tm_setparameter.vi"("error in (no error)"=w629, "Value in"="exp time [s]", "Parameter"=w627, "Handle in"=w628) -> ("error out"=w624:errorcluster, "Handle out"=w625:u32)  [unwired: 6 in]
        n307 = call "tm_setparameter.vi"("error in (no error)"=w624, "Value in"="binning", "Parameter"=w623, "Handle in"=w625) -> ("error out"=w620:errorcluster, "Handle out"=w621:u32)  [unwired: 6 in]
        n308 = call "tm_preparecapture.vi"("error in (no error)"=w620, "Frames"=1, "Capture mode"=w619, "Handle in"=w621) -> ("error out"=w616:errorcluster, "Buffer Info"=w615:T5, "Handle out"=w617:u32)  [unwired: 4 in, 1 out]
        n309 = Unbundle(w615) -> ("height"=w608:u32, "width"=w609:u32)  [unwired: 1 out]
        n310 = call "tm_startcapture_b.vi"("error in (no error)"=w616, "Handle in"=w617) -> ("error out"=w611:errorcluster, "Handle out"=w612:u32)  [unwired: 8 in]
        n311 = property on="live" class="IntGraph (strict)"("XScale.Minimum"=0.0 ("X Scale.Range:Minimum"), "XScale.Maximum"=w608, "YScale.Minimum"=0.0 ("Y Scale.Range:Minimum"), "YScale.Maximum"=w609) -> ()  [unwired: 2 in, 2 out]
        n312 = Initialize Array(u16 0 ("element"), w608, w609) -> (w613:u16[][])
        n313 = To Double Precision Float(number=w613) -> (double precision float=w614:dbl[][])
      }
      frame "close" {
        n314 = Release Queue(queue=w641) -> ()  [unwired: 2 in, 3 out]
      }
    }
  }
  n315 = while {
    tunnel: w10 -> [w650]
    shift-right: [w648] -> _
    shift-left: _ -> [w647]
    shift-right: [w645] -> _
    shift-left: 0 -> [w646]
    shift-right: [w644] -> _
    shift-left: _ -> [w643]
    tunnel: w1 -> [w642]
    stop <- w649 stop-if-true
    # "ISEG"
    n316 = Preview Queue Element(queue=w650, timeout in ms (-1)=w646) -> (element=w654:string)  [unwired: 1 in, 3 out]
    n317 = Match Pattern(string=w654, regular expression=":") -> (before substring=w652:string, after substring=w651:string)  [unwired: 1 in, 2 out]
    n318 = case shown="\"idle\", Default" w652 {
      tunnel: w651 -> [_ w667 _ _ _]
      tunnel: w650 -> [_ w679 w720 w724 w728]
      tunnel: [_ _ _ _ TRUE] -> w649
      tunnel: [w655 w673 w718 w723 w725] -> w648
      tunnel: w647 -> [w657 w677 _ _ w725]
      tunnel: [0 _ _ _ _] -> w645
      tunnel: [w656 w674 T6 {"VISA Resource Name"="", "FP Notation"=FALSE, "Maximum Voltage"=0, "Maximum Current"=0} ("VISA Session Out") w721 w726] -> w644
      tunnel: w643 -> [w658 w678 w719 _ w726]
      tunnel: w642 -> [_ w662 _ _ _]
      frame "idle", Default {
        n319 = local read "Channel (A)"() -> (w660:enum16{"A", "B"})
        n320 = call "iseg NHQ xxx GetActualVoltage.vi"("error in (no error)"=w657, "Channel (A)"=w660, "VISA Session"=w658) -> ("error out"=w655:errorcluster, "Voltage"=→"Actual Voltage":dbl, "VISA Session Out"=w656:T6)  [unwired: 5 in, 1 out]
      }
      frame "set" {
        n321 = local read "Channel (A)"() -> (w670:enum16{"A", "B"})
        n322 = Dequeue Element(queue=w679) -> ()  [unwired: 2 in, 4 out]
        n323 = Match Pattern(string=w667, regular expression=":") -> (before substring=w666:string, after substring=w665:string)  [unwired: 1 in, 2 out]
        n324 = Fract/Exp String To Number(string=w666) -> (number=w669:dbl)  [unwired: 3 in, 1 out]
        n325 = call "iseg NHQ xxx SetNominalVoltage.vi"("error in (no error)"=w677, "Voltage (0 V)"=w669, "Channel (A)"=w670, "VISA Session"=w678) -> ("error out"=w680:errorcluster, "VISA Session Out"=w681:T6)  [unwired: 6 in]
        n326 = Equal?(x=w665, y="wait") -> (x = y?=w663:bool)
        n327 = call "iseg NHQ xxx StartVoltageChange.vi"("error in (no error)"=w680, "Channel (A)"=w670, "VISA Session"=w681) -> ("error out"=w675:errorcluster, "VISA Session Out"=w676:T6)  [unwired: 6 in, 1 out]
        n328 = case shown="True" w663 {
          tunnel: [w683 w693] -> w674
          tunnel: [w682 w685] -> w673
          tunnel: w676 -> [w683 w692]
          tunnel: w675 -> [w682 w691]
          tunnel: w669 -> [_ w690]
          tunnel: "volt_threshold" -> [_ w689]
          tunnel: "volt_timeout" -> [_ w688]
          tunnel: w670 -> [_ w687]
          tunnel: w662 -> [_ w686]
          frame False {
          }
          frame True {
            n329 = Tick Count (ms)() -> (millisecond timer value=w694:u32)
            n330 = while {
              shift-right: [w714] -> w693
              shift-left: w692 -> [w716]
              shift-right: [w700] -> w685
              shift-left: w691 -> [w715]
              tunnel: w687 -> [w713]
              tunnel: w689 -> [w710]
              tunnel: w694 -> [w708]
              tunnel: w688 -> [w706]
              tunnel: w690 -> [w705]
              tunnel: [w695] -> w684
              stop <- w701 stop-if-true
              n331 = Tick Count (ms)() -> (millisecond timer value=w709:u32)
              n332 = call "iseg NHQ xxx GetActualVoltage.vi"("error in (no error)"=w715, "Channel (A)"=w713, "VISA Session"=w716) -> ("error out"=w700:errorcluster, "Voltage"=w703:dbl, "VISA Session Out"=w714:T6)  [unwired: 5 in, 1 out]
              n333 = Absolute Value(x=w703) -> (abs(x)=w704:dbl)
              n334 = Subtract(x=w709, y=w708) -> (x-y=w707:u32)
              n335 = Subtract(x=w704, y=w705) -> (x-y=w712:dbl)
              n336 = local write "Actual Voltage"(w703) -> ()
              n337 = Absolute Value(x=w712) -> (abs(x)=w711:dbl)
              n338 = Greater?(x=w707, y=w706) -> (0:w699:bool)
              n339 = Less?(x=w711, y=w710) -> (x < y?=w702:bool)
              n340 = Or(x=w700, y=w699) -> (x .or. y?=w698:bool)
              n341 = Compound Arithmetic op=OR(w700, w702, w699) -> (w701:bool)
              n342 = Select(t="fail" ("element"), s=w698, f="done" ("element")) -> (s? t:f=w695:string)
            }
            n343 = Enqueue Element(queue=w686, element=w684) -> ()  [unwired: 2 in, 3 out]
          }
        }
      }
      frame "release" {
        n344 = Dequeue Element(queue=w720) -> ()  [unwired: 2 in, 4 out]
        n345 = call "iseg NHQ xxx Close.vi"("VISA session"=w719) -> ("error out"=w718:errorcluster)  [unwired: 14 in]
      }
      frame "init" {
        n346 = Dequeue Element(queue=w724) -> ()  [unwired: 2 in, 4 out]
        n347 = call "iseg NHQ xxx Initialize.vi"("VISA resource name"="VISA ISEG") -> ("VISA Session Out"=w721:T6, "error out"=w723:errorcluster)  [unwired: 13 in]
      }
      frame "close" {
        n348 = Release Queue(queue=w728) -> ()  [unwired: 2 in, 3 out]
      }
    }
    "error out" <- w648
  }
  n349 = while {
    tunnel: w3 -> [w739]
    shift-right: [w729] -> _
    shift-left: errorcluster {"status"=FALSE, "code"=0, "source"=""} ("error constant") -> [w737]
    shift-right: [w731] -> _
    shift-left: _ -> [w736]
    shift-right: [w735] -> _
    shift-left: _ -> [w734]
    tunnel: w1 -> [w733]
    tunnel: w5 -> [w732]
    tunnel: [w732] -> w4
    stop <- w738 stop-if-true
    # "COHERENT"
    n350 = Preview Queue Element(queue=w739, timeout in ms (-1)=w736) -> (element=w743:string)  [unwired: 1 in, 3 out]
    n351 = Match Pattern(string=w743, regular expression=":") -> (before substring=w741:string, after substring=w740:string)  [unwired: 1 in, 2 out]
    n352 = case shown="\"release\"" w741 {
      tunnel: w740 -> [_ _ _ _ _ _]
      tunnel: w739 -> [_ w771 w791 w799 w805 w811]
      tunnel: [_ _ _ _ _ TRUE] -> w738
      tunnel: [w755 w764 w784 w797 w802 w808] -> w729
      tunnel: w737 -> [w757 w768 w786 _ w801 w808]
      tunnel: [0 _ _ _ _ _] -> w730
      tunnel: [w756 w765 w785 0 ("Meter Index") w803 w809] -> w735
      tunnel: w734 -> [w758 w769 w787 w795 _ w809]
      tunnel: w733 -> [_ w767 w790 _ _ _]
      frame "idle", Default {
        n353 = call "CH_LM Measurement Fetch Data.vi"("Meter Index"=w758, "error in (no error)"=w757) -> ("Meter Index"=w756:i32, "Data Array"=w754:T7[], "error out"=w755:errorcluster)  [unwired: 13 in, 2 out]
        n354 = property on="power history" class="WFChart (strict)"() -> ("History Data"=w752:dbl[])  [unwired: 2 in, 2 out]
        n355 = Index Array(array=w754) -> (element=w753:T7)  [unwired: 1 in]
        n356 = Unbundle By Name(w753) -> ("Value"=w746:sgl)
        n357 = call <vilib>:"Std Deviation and Variance.vi"("X"=w752) -> ("mean"=w747:dbl, "standard deviation"=w750:dbl)  [unwired: 1 in, 1 out]
        n358 = Divide(x=w750, y=w747) -> (x/y=w749:dbl)
        n359 = local write "power history"(w746) -> ()
        n360 = local write "laser power"(w746) -> ()
        n361 = Multiply(x=w749, y=100.0) -> (x*y=→"power noise-o-meter":dbl)
      }
      frame "start" {
        n362 = Dequeue Element(queue=w771) -> (queue out=w770:refnum<queue>)  [unwired: 2 in, 3 out]
        n363 = while {
          tunnel: w770 -> [w780]
          tunnel: w769 -> [w777]
          tunnel: w768 -> [w776]
          tunnel: [w772] -> w766 mode=indexing
          tunnel: [w775] -> w765
          tunnel: [w774] -> w764
          stop <- w781 continue-if-true
          n364 = call "CH_LM Measurement Fetch Data.vi"("Meter Index"=w777, "error in (no error)"=w776) -> ("Meter Index"=w775:i32, "Data Array"=w779:T7[], "error out"=w774:errorcluster)  [unwired: 13 in, 2 out]
          n365 = Index Array(array=w779) -> (element=w778:T7)  [unwired: 1 in]
          n366 = Dequeue Element(queue=w780, timeout in ms (-1)=0) -> (element=w783:string)  [unwired: 1 in, 3 out]
          n367 = Equal?(x=w783, y="") -> (x = y?=w781:bool)
          n368 = Unbundle By Name(w778) -> ("Value"=w772:sgl)
          n369 = local write "laser power"(w772) -> ()
        }
        n370 = call <vilib>:"Std Deviation and Variance.vi"("X"=w766) -> ("mean"=w762:dbl, "standard deviation"=w761:dbl)  [unwired: 1 in, 1 out]
        n371 = Format Into String(format string="%.6e;%.6e", w762, w761) -> (resulting string=w760:string)  [unwired: 2 in, 1 out]
        n372 = Enqueue Element(queue=w767, element=w760) -> ()  [unwired: 2 in, 3 out]
      }
      frame "snap" {
        n373 = Dequeue Element(queue=w791) -> ()  [unwired: 2 in, 4 out]
        n374 = call "CH_LM Measurement Fetch Data.vi"("Meter Index"=w787, "error in (no error)"=w786) -> ("Meter Index"=w785:i32, "Data Array"=w793:T7[], "error out"=w784:errorcluster)  [unwired: 13 in, 2 out]
        n375 = Index Array(array=w793) -> (element=w792:T7)  [unwired: 1 in]
        n376 = Unbundle By Name(w792) -> ("Value"=w788:sgl)
        n377 = local write "laser power"(w788) -> ()
        n378 = Format Into String(format string="%.6e", w788) -> (resulting string=w789:string)  [unwired: 2 in, 1 out]
        n379 = Enqueue Element(queue=w790, element=w789) -> ()  [unwired: 2 in, 3 out]
      }
      frame "release" {
        n380 = Dequeue Element(queue=w799) -> ()  [unwired: 2 in, 4 out]
        n381 = call "CH_LM Measurement Abort.vi"("Meter Index"=w795) -> ("Meter Index"=w796:i32)  [unwired: 16 in, 2 out]
        n382 = call "CH_LM Close.vi"("Meter Index"=w796) -> ("error out"=w797:errorcluster)  [unwired: 16 in, 2 out]
      }
      frame "init" {
        n383 = Dequeue Element(queue=w805) -> ()  [unwired: 2 in, 4 out]
        n384 = flat-sequence {
          tunnel: w801 -> [w807]
          tunnel: [w807] -> w800
          frame #0 {
            n385 = Wait (ms)(milliseconds to wait=u32 1000) -> ()  [unwired: 1 out]
          }
        }
        n386 = call "CH_LM Measurement Initiate.vi"("Meter Index"=0, "error in (no error)"=w800) -> ("Meter Index"=w803:i32, "error out"=w802:errorcluster)  [unwired: 15 in, 1 out]
      }
      frame "close" {
        n387 = Release Queue(queue=w811) -> ()  [unwired: 2 in, 3 out]
      }
    }
    "coherent" <- w729
    n388 = case shown="No Error" w729 {
      tunnel: [w744 -1] -> w731
      tunnel: w730 -> [w744 _]
      frame No Error {
      }
      frame Error {
      }
    }
  }
  n389 = Set Occurrence(w4) -> ()
